vi "Q14070-Z040轴向间隙测试台1.vi"() -> ()   [LabVIEW 2013]
uses:
  <vilib>/printing/EasyPrintingControls.llb/report_type.ctl
  <vilib>/printing/EasyPrintingControls.llb/contents.ctl
  <vilib>/Utility/NIReport.llb/NI_report.lvclass
  <vilib>/Utility/file.llb/Write To Spreadsheet File (DBL).vi
  <vilib>/printing/EasyPrinting.llb/Easy Print VI Panel or Documentation (path).vi
  PCI8622_32.dll
  <vilib>/Utility/NIReport.llb/NI_ReportGenerationCore.lvlib
panel:
  in  "循环次数":u16
  out "左最大间隙值(mm)":dbl format="%#.6f"
  out "右最大间隙值(mm)":dbl format="%#.6f"
  out "旋转左极限位(mm)":dbl=-40.0
  out "旋转右极限位(mm)":dbl=60.0
  out "输入轴快进位置(mm)":dbl=-40.0
  out "输入轴初始位置(mm)":dbl=60.0
  out "输入轴最终位置（mm)":dbl format="%#.3f"
  out "左右基准":dbl=-40.0
  in  "进给速度":dbl=10.0
  in  "旋转速度":dbl=10.0
  out "DeviceHandle":u32
  out "输入轴电机慢进位置3":dbl format="%#.3f"
  out "输入轴电机慢进位置2":dbl format="%#.3f"
  out "旋转轴伺服位置":dbl=10000.0 format="%#.2f"
  out "复位按钮":bool=TRUE
  out "报警工步号":dbl
  out "报警信息":string
  out "输入轴伺服位置":dbl=10000.0 format="%#.1f"
  out "力矩（nm)":dbl format="%#.2f"
  out "位移(mm)":dbl format="%#.3f"
  in  "员工权限":bool
  out "测试操作状态":string
  out "测试 工步号":dbl
  out "通讯状态":bool
  in  "停止":bool
  out "流水线操作状态":string
  in  "流水线工步号":dbl
  in  "联线按钮":bool
  in  "选项卡控件 2":enum32{"间隙曲线", "手动", "传感器校验", "参数查询"}(tab)
  out "检测扭矩(NM)":dbl format="%#.1f"
  out "轴向间隙值(mm)":dbl format="%#.3f"
  out "本序完成":bool
  out "上序合格":bool
  out "上序完成":bool
  out "本序合格":bool
  out "间隙合格标准值(mm)":dbl=0.2
  out "换向扭矩(NM)":dbl format="%#.1f"
  out "XY图":cluster{dbl[], dbl[]}[](graph)
  in  "扳手无效":bool
  out "流水线气缸下限":bool
  out "流水线气缸上限":bool
  out "下工位检测":bool
  out "本工位检测":bool
  out "上工位检测":bool
  in  "M顶升气缸上升":bool
  in  "M顶升气缸下降":bool
  in  "M本阻挡器":bool
  in  "M上阻挡器":bool
  in  "电机回零":bool
  in  "电机下降":bool
  in  "电机上升":bool
  in  "左旋":bool
  in  "右旋":bool
  in  "扭矩传感器零点偏移":dbl format="%#.2f"
  in  "扭矩传感器比例偏移":dbl=1.0 format="%#.2f"
  in  "位移传感器零点偏移":dbl format="%#.2f"
  in  "位移传感器比例偏移":dbl=1.0 format="%#.2f"
  in  "传感器参数保存":bool
  in  "参数查询":bool
  in  "参数列表":string[][](table)
  in  "员工ID":string
  out "员工姓名":string
  in  "型号选择":u16(ring) items=["J706", "J709"]
  in  "参数加载":bool
  out "产品ID":string
  out "轴向间隙比例系数":dbl=1.0 format="%#_2f"
  out "error out 2":errorcluster
  out "输入轴电机快进速度":dbl format="%#.1f"
  out "输入轴电机慢进速度":dbl format="%#.3f"
  out "旋转电机速度":dbl=5.0 format="%#.3f"
  out "ADODB._Connection Out":refnum<k7>
  out "error out 3":errorcluster
  out "error out":errorcluster
  out "急停按钮":bool=TRUE
  out "芯片ID":string
  out "旋转轴AxisHandle OUT":u32
  out "FGCS":string
  out "RFID读取完成":bool
  out "RFID读取触发":bool
  out "Z040 RFID":string="A001"
  out "KSJJ":string
  out "ReturnValue 3":u32
  out "ReturnValue":u32
  out "输入轴AxisHandle OUT":u32
  out "产品选型":dbl
  # "Q14070-Z040  齿轮轴轴向间隙测试台"
  # "Q14070机械转向器装配线"
  # "Copying (C) 2015 湖北唯思凌科装备制造有限公司 版权所有"
  # "≤"
  # "传感器校验区"
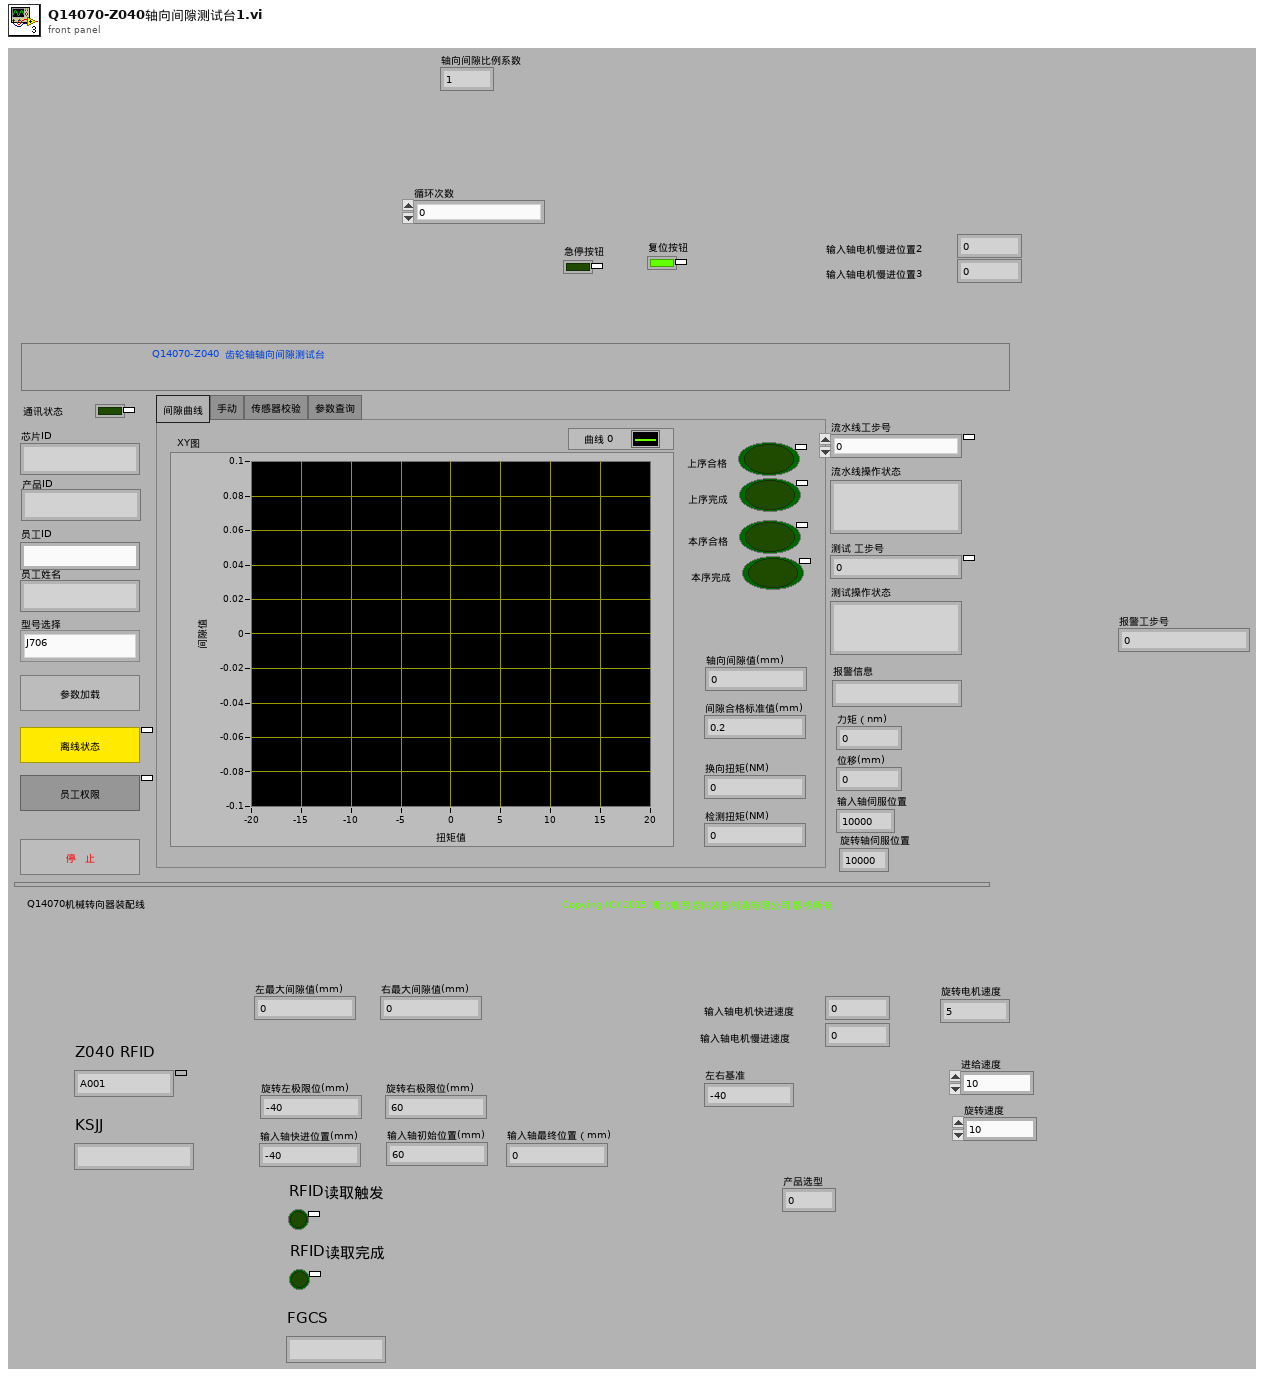
[diagram p1: front panel]
types:
  T1 = typedef "NI_ReportGenerationCore.lvlib/contents.ctl" = u16
  T2 = typedef "NI_ReportGenerationCore.lvlib/report_type.ctl" = u16
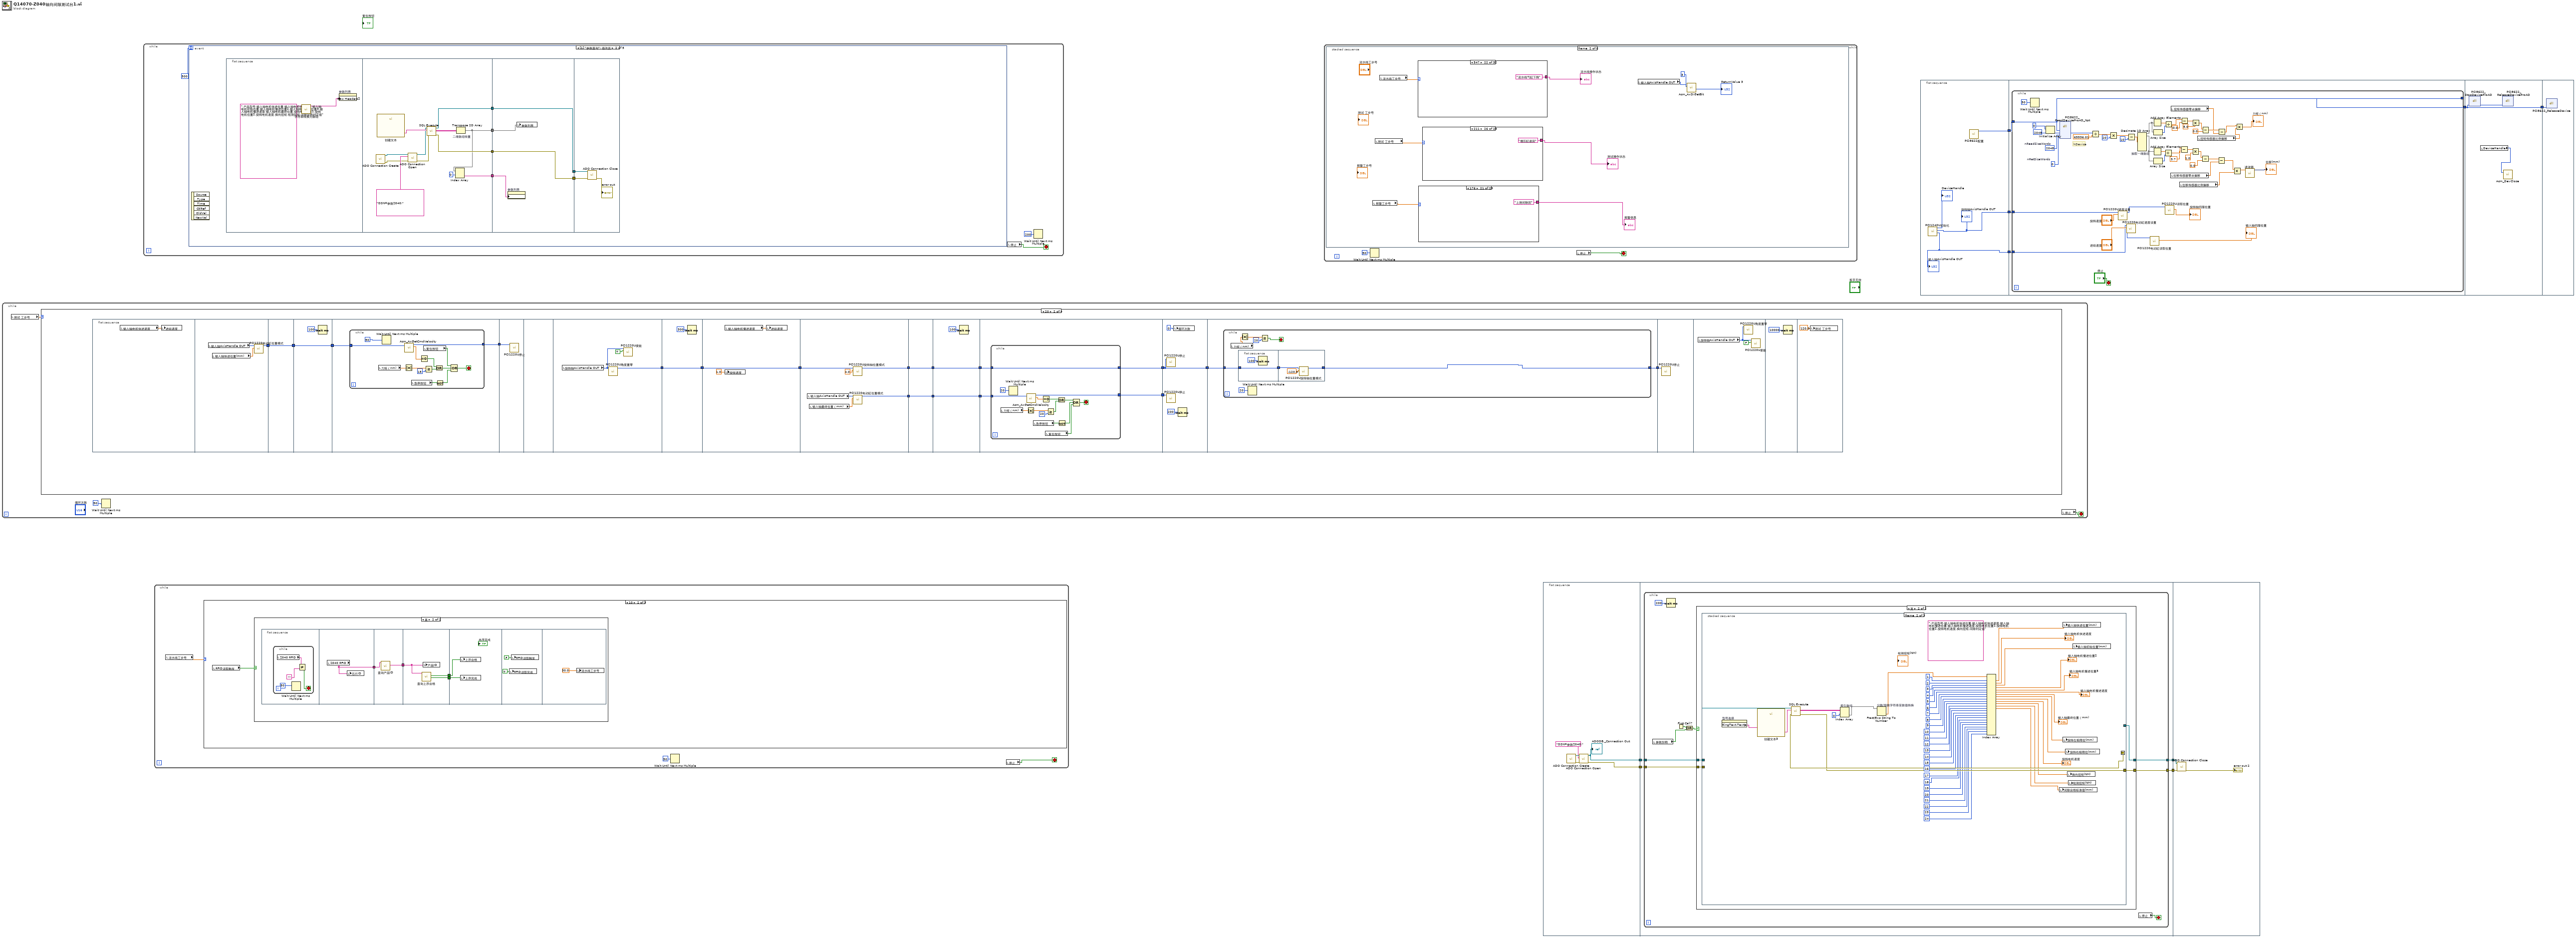
[diagram p0: block diagram]
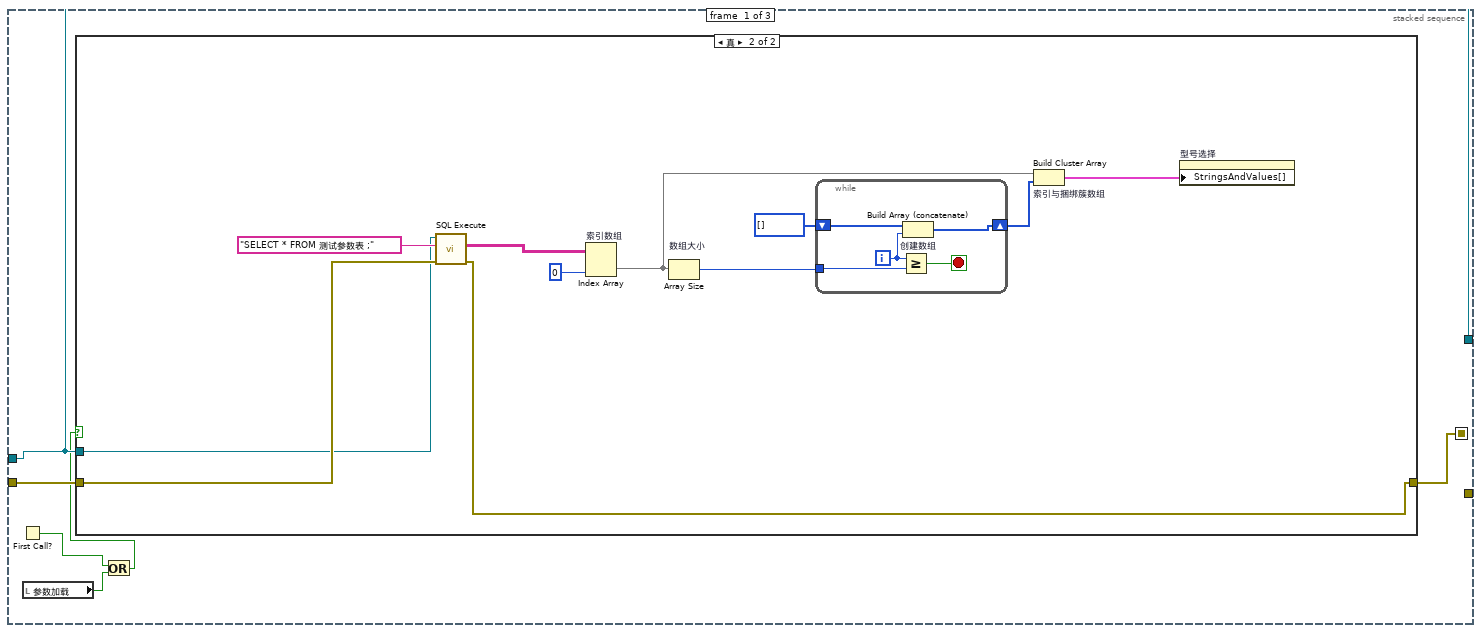
[diagram p3: hidden frame]
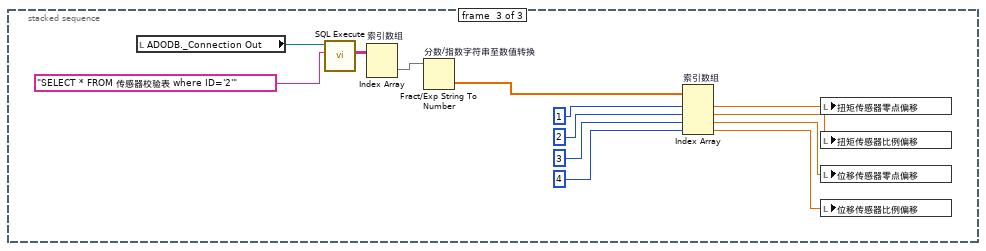
[diagram p5: hidden frame]
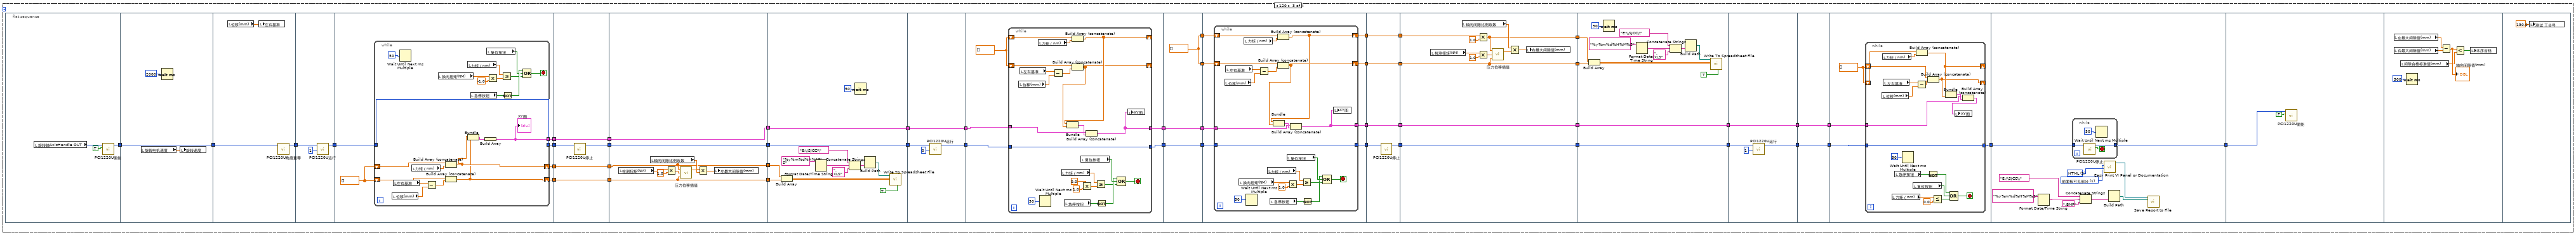
[diagram p7: hidden frame]
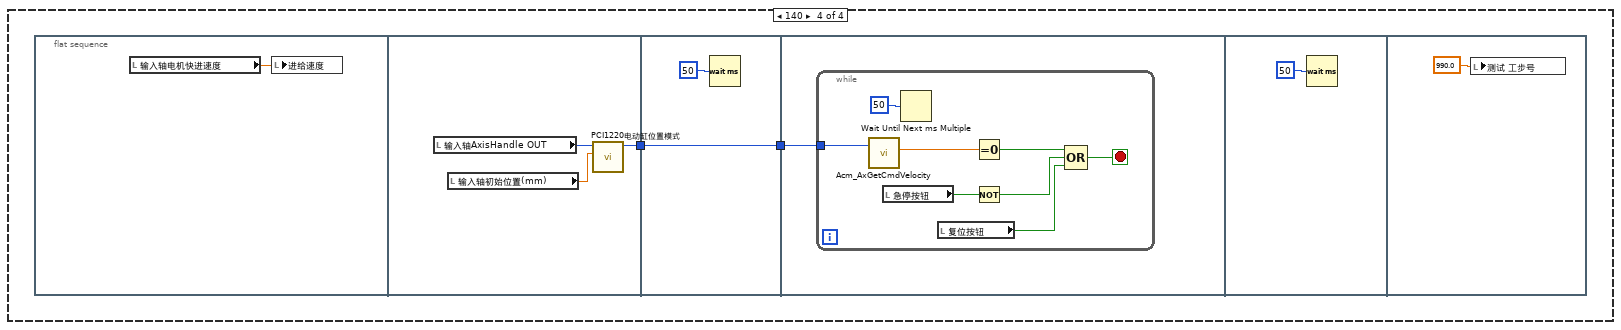
[diagram p8: hidden frame]
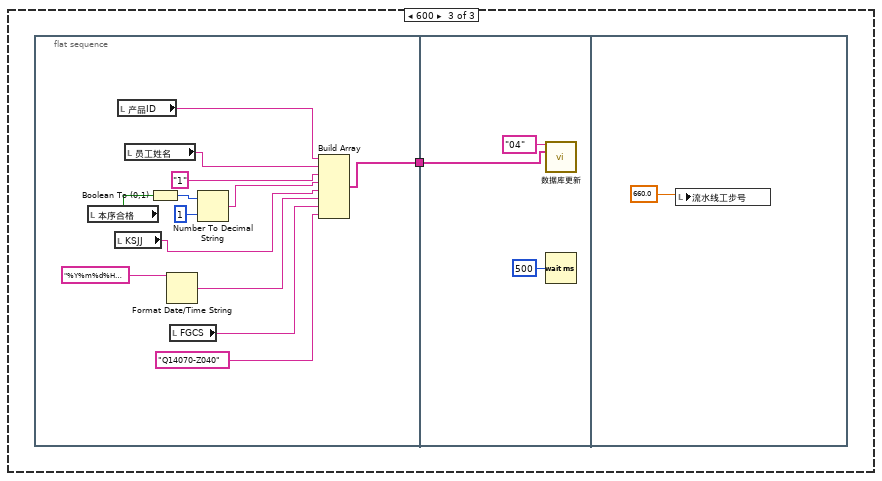
[diagram p11: hidden frame]
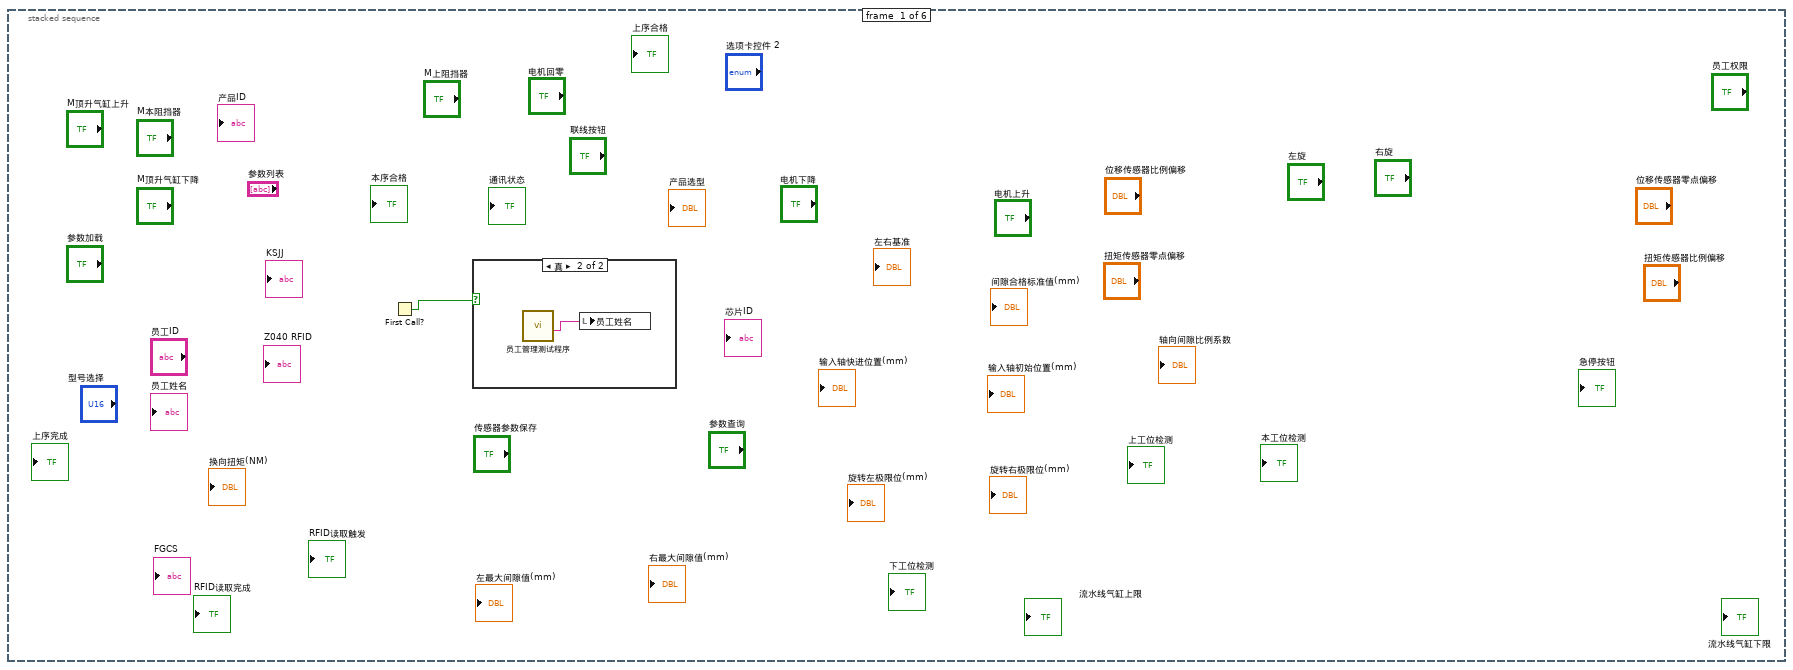
[diagram p12: hidden frame]
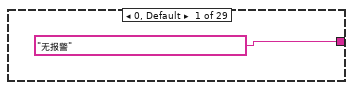
[diagram p14: hidden frame]
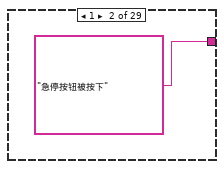
[diagram p15: hidden frame]
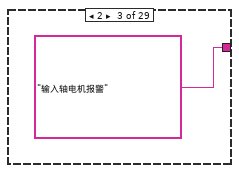
[diagram p16: hidden frame]
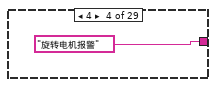
[diagram p17: hidden frame]
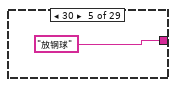
[diagram p18: hidden frame]
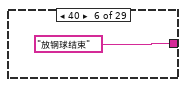
[diagram p19: hidden frame]
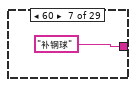
[diagram p20: hidden frame]
diagram:
  n1 = while {
    stop <- w10 stop-if-true
    n2 = local read "测试 工步号"() -> (w12:dbl)
    n3 = case shown="20" w12 {
      frame 0, Default {
      }
      frame 20 {
        n4 = flat-sequence {
          tunnel: [w33] -> w23
          tunnel: [w34] -> w27
          tunnel: w23 -> [w34]
          tunnel: w27 -> [w36]
          tunnel: [w36] -> w26
          tunnel: w26 -> [w38]
          tunnel: [w37] -> w29
          tunnel: w29 -> [w53]
          tunnel: [w55] -> w17
          tunnel: w17 -> [w58]
          tunnel: [w58] -> w16
          tunnel: w16 -> [w61]
          tunnel: [w61] -> w15
          tunnel: [w65] -> w22
          tunnel: w15 -> [w64]
          tunnel: [w62] -> w19
          tunnel: [w68] -> w25
          tunnel: w22 -> [w68]
          tunnel: [w69] -> w21
          tunnel: w19 -> [w69]
          tunnel: w25 -> [w72]
          tunnel: [w72] -> w24
          tunnel: w21 -> [w70]
          tunnel: [w70] -> w20
          tunnel: w24 -> [w76]
          tunnel: [w75] -> w28
          tunnel: w20 -> [w74]
          tunnel: [w73] -> w18
          tunnel: w28 -> [w95]
          tunnel: w18 -> [w93]
          tunnel: [w93] -> w14
          tunnel: w14 -> [w97]
          tunnel: [w96] -> w13
          tunnel: w13 -> [w111]
          frame #0 {
            n5 = local read "输入轴电机快进速度"() -> (w30:dbl)
            n6 = local write "进给速度"(w30) -> ()
          }
          frame #1 {
            n7 = local read "输入轴AxisHandle OUT"() -> (w31:u32)
            n8 = local read "输入轴快进位置(mm)"() -> (w32:dbl)
            n9 = call "PCI1220电动缸位置模式 .vi"("Distance"=w32, "AxisHandle IN"=w31) -> ("AxisHandle OUT"=w33:u32)  [unwired: 8 in, 1 out]
          }
          frame #2 {
          }
          frame #3 {
            n10 = Wait (ms)(milliseconds to wait=u32 100 ("等待时间（毫秒）")) -> ()  [unwired: 1 out]
          }
          frame #4 {
            n11 = while {
              tunnel: w38 -> [w49]
              tunnel: [w50] -> w37
              stop <- w40 stop-if-true
              n12 = local read "力矩（nm)"() -> (w47:dbl)
              n13 = Wait Until Next ms Multiple(millisecond multiple=u32 50 ("毫秒倍数")) -> ()  [unwired: 1 out]
              n14 = Absolute Value(x=w47) -> (abs(x)=w46:dbl)
              n15 = call <userlib>:"Acm_AxGetCmdVelocity.vi"("AxisHandle"=w49) -> ("Velocity"=w51:dbl, "AxisHandle"=w50:u32)  [unwired: 1 in, 2 out]
              n16 = local read "急停按钮"() -> (w43:bool)
              n17 = Equal To 0?(x=w51) -> (x = 0?=w48:bool)
              n18 = local read "复位按钮"() -> (w39:bool)
              n19 = Greater Or Equal?(x=w46, y=15) -> (x >= y?=w44:bool)
              n20 = Or(x=w48, y=w44) -> (x .or. y?=w42:bool)
              n21 = Not(x=w43) -> (.not. x?=w41:bool)
              n22 = Compound Arithmetic op=OR(w39, w42, w41) -> (w40:bool)
            }
          }
          frame #5 {
            n23 = call "PCI1220U停止.vi"("AxisHandle IN"=w53) -> ()  [unwired: 9 in, 2 out]
          }
          frame #6 {
          }
          frame #7 {
            n24 = local read "旋转轴AxisHandle OUT"() -> (w56:u32)
            n25 = call "PCI1220U角度置零.vi"("AxisHandle IN"=w56) -> ("AxisHandle OUT"=w55:u32)  [unwired: 10 in]
            n26 = call "PCI1220U使能.vi"("使能"=TRUE, "AxisHandle IN"=w56) -> ()  [unwired: 9 in, 1 out]
          }
          frame #8 {
            n27 = Wait (ms)(milliseconds to wait=u32 300 ("毫秒倍数")) -> ()  [unwired: 1 out]
          }
          frame #9 {
            n28 = local write "旋转速度"(1.0 ("旋转速度")) -> ()
            n29 = local read "输入轴电机慢进速度"() -> (w59:dbl)
            n30 = local write "进给速度"(w59) -> ()
          }
          frame #10 {
            n31 = local read "输入轴AxisHandle OUT"() -> (w67:u32)
            n32 = local read "输入轴最终位置（mm)"() -> (w66:dbl)
            n33 = call "PCI1220U旋转轴位置模式.vi"("Distance"=4.0, "AxisHandle IN"=w64) -> ("AxisHandle OUT"=w62:u32)  [unwired: 8 in, 1 out]
            n34 = call "PCI1220电动缸位置模式 .vi"("Distance"=w66, "AxisHandle IN"=w67) -> ("AxisHandle OUT"=w65:u32)  [unwired: 8 in, 1 out]
          }
          frame #11 {
          }
          frame #12 {
            n35 = Wait (ms)(milliseconds to wait=u32 100 ("等待时间（毫秒）")) -> ()  [unwired: 1 out]
          }
          frame #13 {
            n36 = while {
              tunnel: w76 -> [w90]
              tunnel: [w88] -> w75
              tunnel: w74 -> [w77]
              tunnel: [w77] -> w73
              stop <- w79 stop-if-true
              n37 = local read "力矩（nm)"() -> (w85:dbl)
              n38 = Wait Until Next ms Multiple(millisecond multiple=u32 20 ("毫秒倍数")) -> ()  [unwired: 1 out]
              n39 = Absolute Value(x=w85) -> (abs(x)=w86:dbl)
              n40 = call <userlib>:"Acm_AxGetCmdVelocity.vi"("AxisHandle"=w90) -> ("Velocity"=w89:dbl, "AxisHandle"=w88:u32)  [unwired: 1 in, 2 out]
              n41 = local read "急停按钮"() -> (w83:bool)
              n42 = Equal To 0?(x=w89) -> (x = 0?=w78:bool)
              n43 = local read "复位按钮"() -> (w80:bool)
              n44 = Greater Or Equal?(x=w86, y=20) -> (x >= y?=w84:bool)
              n45 = Or(x=w78, y=w84) -> (x .or. y?=w82:bool)
              n46 = Not(x=w83) -> (.not. x?=w81:bool)
              n47 = Compound Arithmetic op=OR(w82, w81, w80) -> (w79:bool)
            }
          }
          frame #14 {
            n48 = call "PCI1220U停止.vi"("AxisHandle IN"=w93) -> ()  [unwired: 9 in, 2 out]
            n49 = call "PCI1220U停止.vi"("AxisHandle IN"=w95) -> ()  [unwired: 9 in, 2 out]
            n50 = local write "循环次数"(u16 0 ("循环次数")) -> ()
            n51 = Wait (ms)(milliseconds to wait=u32 200 ("毫秒计时值")) -> ()  [unwired: 1 out]
          }
          frame #15 {
            n52 = while {
              tunnel: w97 -> [w99]
              tunnel: [w100] -> w96
              stop <- w102 stop-if-true
              n53 = local read "力矩（nm)"() -> (w101:dbl)
              n54 = flat-sequence {
                tunnel: w99 -> [w106]
                tunnel: [w106] -> w98
                tunnel: [w109] -> w100
                tunnel: w98 -> [w108]
                frame #0 {
                  n55 = Wait (ms)(milliseconds to wait=u32 100 ("等待时间（毫秒）")) -> ()  [unwired: 1 out]
                }
                frame #1 {
                  n56 = call "PCI1220U旋转轴位置模式.vi"("Distance"=-120.0, "AxisHandle IN"=w108) -> ("AxisHandle OUT"=w109:u32)  [unwired: 8 in, 1 out]
                }
              }
              n57 = Absolute Value(x=w101) -> (abs(x)=w103:dbl)
              n58 = Wait Until Next ms Multiple(millisecond multiple=u32 20 ("毫秒倍数")) -> ()  [unwired: 1 out]
              n59 = Greater Or Equal?(x=w103, y=20) -> (x >= y?=w102:bool)
            }
          }
          frame #16 {
            n60 = call "PCI1220U停止.vi"("AxisHandle IN"=w111) -> ()  [unwired: 9 in, 2 out]
          }
          frame #17 {
            n61 = local read "旋转轴AxisHandle OUT"() -> (w113:u32)
            n62 = call "PCI1220U角度置零.vi"("AxisHandle IN"=w113) -> ()  [unwired: 10 in, 1 out]
            n63 = call "PCI1220U使能.vi"("使能"=FALSE, "AxisHandle IN"=w113) -> ()  [unwired: 9 in, 1 out]
          }
          frame #18 {
            n64 = Wait (ms)(milliseconds to wait=u32 10000 ("等待时间（毫秒）")) -> ()  [unwired: 1 out]
          }
          frame #19 {
            n65 = local write "测试 工步号"(120.0 ("流水线工步号")) -> ()
          }
        }
      }
      frame 120 {
        n66 = flat-sequence {
          tunnel: [w162] -> w150
          tunnel: [w167] -> w151
          tunnel: w150 -> [w167]
          tunnel: w151 -> [w170]
          tunnel: [w169] -> w131
          tunnel: w131 -> [w172]
          tunnel: [w171] -> w139
          tunnel: w139 -> [w179]
          tunnel: [w178] -> w161
          tunnel: [w177] -> w160
          tunnel: [w176] -> w149
          tunnel: [w175] -> w128
          tunnel: w161 -> [w205]
          tunnel: w160 -> [w204]
          tunnel: [w204] -> w159
          tunnel: [w203] -> w158
          tunnel: [w202] -> w157
          tunnel: w149 -> [w203]
          tunnel: w128 -> [w201]
          tunnel: [w201] -> w127
          tunnel: w159 -> [w207]
          tunnel: w158 -> [w208]
          tunnel: w157 -> [w215]
          tunnel: [w215] -> w135
          tunnel: [w208] -> w133
          tunnel: [w207] -> w132
          tunnel: w127 -> [w206]
          tunnel: [w206] -> w126
          tunnel: w135 -> [w228]
          tunnel: [w228] -> w134
          tunnel: w133 -> [w220]
          tunnel: w132 -> [w219]
          tunnel: [w217] -> w130
          tunnel: w126 -> [w217]
          tunnel: w134 -> [w231]
          tunnel: [w230] -> w125
          tunnel: w130 -> [w229]
          tunnel: [w229] -> w123
          tunnel: w125 -> [w237]
          tunnel: [w234] -> w124
          tunnel: w123 -> [w236]
          tunnel: [w235] -> w122
          tunnel: [w262] -> w153
          tunnel: [w260] -> w152
          tunnel: [w260] -> w142
          tunnel: w124 -> [w262]
          tunnel: [w261] -> w129
          tunnel: w122 -> [w261]
          tunnel: w153 -> [w270]
          tunnel: w152 -> [w268]
          tunnel: [w269] -> w156
          tunnel: [w266] -> w155
          tunnel: [w265] -> w154
          tunnel: w142 -> [w267]
          tunnel: w129 -> [w264]
          tunnel: [w263] -> w121
          tunnel: w156 -> [w297]
          tunnel: w155 -> [w296]
          tunnel: [w296] -> w138
          tunnel: w154 -> [w295]
          tunnel: [w295] -> w137
          tunnel: [w294] -> w136
          tunnel: w121 -> [w293]
          tunnel: [w293] -> w120
          tunnel: w138 -> [w302]
          tunnel: w137 -> [w304]
          tunnel: [w307] -> w147
          tunnel: w136 -> [w307]
          tunnel: [w303] -> w141
          tunnel: [w302] -> w140
          tunnel: w120 -> [w298]
          tunnel: [w298] -> w119
          tunnel: [w322] -> w148
          tunnel: w147 -> [w322]
          tunnel: w141 -> [w315]
          tunnel: w140 -> [w314]
          tunnel: w119 -> [w310]
          tunnel: [w310] -> w118
          tunnel: w148 -> [w325]
          tunnel: [w324] -> w145
          tunnel: w118 -> [w323]
          tunnel: [w323] -> w117
          tunnel: [w328] -> w146
          tunnel: w145 -> [w328]
          tunnel: w117 -> [w327]
          tunnel: [w327] -> w116
          tunnel: w146 -> [w332]
          tunnel: [w331] -> w144
          tunnel: w116 -> [w329]
          tunnel: w144 -> [w363]
          tunnel: [w362] -> w143
          tunnel: w143 -> [w368]
          frame #0 {
            n67 = local read "旋转轴AxisHandle OUT"() -> (w164:u32)
            n68 = call "PCI1220U使能.vi"("使能"=TRUE, "AxisHandle IN"=w164) -> ("AxisHandle OUT"=w162:u32)  [unwired: 9 in]
          }
          frame #1 {
            n69 = local read "旋转电机速度"() -> (w166:dbl)
            n70 = Wait (ms)(milliseconds to wait=u32 2000 ("毫秒倍数")) -> ()  [unwired: 1 out]
            n71 = local write "旋转速度"(w166) -> ()
          }
          frame #2 {
            n72 = local read "位移(mm)"() -> (w168:dbl)
            n73 = local write "左右基准"(w168) -> ()
            n74 = call "PCI1220U角度置零.vi"("AxisHandle IN"=w170) -> ("AxisHandle OUT"=w169:u32)  [unwired: 10 in]
          }
          frame #3 {
            n75 = call "PCI1220U运行.vi"("方向"=u16 1, "AxisHandle IN"=w172) -> ("AxisHandle OUT"=w171:u32)  [unwired: 9 in]
          }
          frame #4 {
            w174 = dbl[] [] ("添加的数组")
            n76 = while {
              tunnel: w179 -> [w193]
              tunnel: [w193] -> w178
              shift-right: [w182] -> w176
              shift-left: w174 -> [w183]
              shift-right: [w181] -> w177
              shift-left: w174 -> [w187]
              tunnel: [w180] -> w175
              stop <- w188 stop-if-true
              n77 = local read "位移(mm)"() -> (w186:dbl)
              n78 = local read "左右基准"() -> (w185:dbl)
              n79 = Wait Until Next ms Multiple(millisecond multiple=u32 50 ("毫秒倍数")) -> ()  [unwired: 1 out]
              n80 = local read "力矩（nm)"() -> (w200:dbl)
              n81 = Subtract(x=w185, y=w186) -> (x-y=w198:dbl)
              n82 = local read "换向扭矩(NM)"() -> (w197:dbl)
              n83 = Build Array (concatenate)(w183, w200) -> (w182:dbl[])
              n84 = Build Array (concatenate)(w187, w198) -> (w181:dbl[])
              n85 = Bundle(w182, w181) -> (w184:cluster{dbl[], dbl[]})  [unwired: 1 in]
              n86 = local read "力矩（nm)"() -> (w195:dbl)
              n87 = local read "急停按钮"() -> (w192:bool)
              n88 = Build Array(w184) -> (w180:cluster{dbl[], dbl[]}[])
              "XY图" <- w180
              n89 = local read "复位按钮"() -> (w190:bool)
              n90 = Multiply(x=w197, y=-1.0) -> (x*y=w194:dbl)
              n91 = Less Or Equal?(x=w195, y=w194) -> (x <= y?=w189:bool)
              n92 = Not(x=w192) -> (.not. x?=w191:bool)
              n93 = Compound Arithmetic op=OR(w191, w190, w189) -> (w188:bool)
            }
          }
          frame #5 {
            n94 = call "PCI1220U停止.vi"("AxisHandle IN"=w205) -> ("AxisHandle OUT"=w202:u32)  [unwired: 9 in, 1 out]
          }
          frame #6 {
            n95 = local read "检测扭矩(NM)"() -> (w209:dbl)
            n96 = local read "轴向间隙比例系数"() -> (w212:dbl)
            n97 = Multiply(x=w209, y=1.0) -> (x*y=w211:dbl)
            n98 = call "压力位移插值.vi"("压力数组"=w207, "监控点位移"=w211, "位移数组"=w208) -> ("监控点压力"=w213:dbl)  [unwired: 2 in]
            n99 = Multiply(x=w212, y=w213) -> (x*y=w214:dbl)
            n100 = local write "左最大间隙值(mm)"(w214) -> ()
          }
          frame #7 {
            n101 = Build Array(w220, w219) -> (w218:dbl[][])
            n102 = Format Date/Time String(time format string (%c)="%y%m%d%H%M%S" ("时间格式字符串(%c)")) -> (date/time string=w227:string)  [unwired: 2 in]
            n103 = Concatenate Strings("E:\\SJCC\\" ("时间格式字符串(%c)"), w227, ".XLS") -> (w222:string)
            n104 = Wait (ms)(milliseconds to wait=u32 50 ("等待时间（毫秒）")) -> ()  [unwired: 1 out]
            n105 = Build Path(name or relative path=w222) -> (appended path=w223:path)  [unwired: 1 in]
            n106 = call-poly <vilib>:"Write To Spreadsheet File.vi"("transpose? (no:F)"=TRUE, "2D data"=w218, "file path (dialog if empty)"=w223) -> ()  [unwired: 5 in, 1 out]
          }
          frame #8 {
            n107 = call "PCI1220U运行.vi"("方向"=u16 0, "AxisHandle IN"=w231) -> ("AxisHandle OUT"=w230:u32)  [unwired: 9 in]
          }
          frame #9 {
            w233 = dbl[] [] ("添加的数组")
            n108 = while {
              tunnel: w237 -> [w254]
              tunnel: [w254] -> w234
              shift-right: [w243] -> _
              shift-left: w233 -> [w248]
              shift-right: [w242] -> _
              shift-left: w233 -> [w247]
              tunnel: w236 -> [w239]
              tunnel: [w241] -> w235
              stop <- w249 stop-if-true
              n109 = local read "位移(mm)"() -> (w245:dbl)
              n110 = local read "左右基准"() -> (w244:dbl)
              n111 = local read "力矩（nm)"() -> (w259:dbl)
              n112 = Wait Until Next ms Multiple(millisecond multiple=u32 50 ("毫秒倍数")) -> ()  [unwired: 1 out]
              n113 = Subtract(x=w244, y=w245) -> (x-y=w246:dbl)
              n114 = local read "力矩（nm)"() -> (w257:dbl)
              n115 = local read "急停按钮"() -> (w251:bool)
              n116 = Build Array (concatenate)(w248, w259) -> (w243:dbl[])
              n117 = Build Array (concatenate)(w247, w246) -> (w242:dbl[])
              n118 = Bundle(w243, w242) -> (w238:cluster{dbl[], dbl[]})  [unwired: 1 in]
              n119 = local read "复位按钮"() -> (w253:bool)
              n120 = Multiply(x=0.0, y=1.0) -> (x*y=w255:dbl)
              n121 = Build Array (concatenate)(w239, w238) -> (w241:cluster{dbl[], dbl[]}[])
              n122 = Greater Or Equal?(x=w257, y=w255) -> (x >= y?=w250:bool)
              n123 = Not(x=w251) -> (.not. x?=w252:bool)
              n124 = Compound Arithmetic op=OR(w252, w253, w250) -> (w249:bool)
              n125 = local write "XY图"(w241) -> ()
            }
          }
          frame #10 {
            w260 = dbl[] [] ("添加的数组")
          }
          frame #11 {
            n126 = while {
              tunnel: w270 -> [w286]
              tunnel: [w286] -> w269
              shift-right: [w275] -> w265
              shift-left: w268 -> [w280]
              shift-right: [w274] -> w266
              shift-left: w267 -> [w279]
              tunnel: w264 -> [w271]
              tunnel: [w273] -> w263
              stop <- w281 stop-if-true
              n127 = local read "位移(mm)"() -> (w277:dbl)
              n128 = local read "左右基准"() -> (w276:dbl)
              n129 = local read "换向扭矩(NM)"() -> (w289:dbl)
              n130 = local read "力矩（nm)"() -> (w292:dbl)
              n131 = Wait Until Next ms Multiple(millisecond multiple=u32 50 ("毫秒倍数")) -> ()  [unwired: 1 out]
              n132 = Subtract(x=w276, y=w277) -> (x-y=w278:dbl)
              n133 = local read "力矩（nm)"() -> (w290:dbl)
              n134 = local read "急停按钮"() -> (w283:bool)
              n135 = Build Array (concatenate)(w280, w292) -> (w275:dbl[])
              n136 = Build Array (concatenate)(w279, w278) -> (w274:dbl[])
              n137 = Bundle(w275, w274) -> (w272:cluster{dbl[], dbl[]})  [unwired: 1 in]
              n138 = local read "复位按钮"() -> (w285:bool)
              n139 = Multiply(x=w289, y=1.0) -> (x*y=w287:dbl)
              n140 = Build Array (concatenate)(w271, w272) -> (w273:cluster{dbl[], dbl[]}[])
              n141 = Greater Or Equal?(x=w290, y=w287) -> (x >= y?=w282:bool)
              n142 = Not(x=w283) -> (.not. x?=w284:bool)
              n143 = Compound Arithmetic op=OR(w284, w285, w282) -> (w281:bool)
              n144 = local write "XY图"(w273) -> ()
            }
          }
          frame #12 {
            n145 = call "PCI1220U停止.vi"("AxisHandle IN"=w297) -> ("AxisHandle OUT"=w294:u32)  [unwired: 9 in, 1 out]
          }
          frame #13 {
            n146 = local read "检测扭矩(NM)"() -> (w301:dbl)
            n147 = local read "轴向间隙比例系数"() -> (w309:dbl)
            n148 = Multiply(x=w304, y=1.0) -> (x*y=w303:dbl[])
            n149 = Multiply(x=w301, y=1.0) -> (x*y=w300:dbl)
            n150 = call "压力位移插值.vi"("压力数组"=w302, "监控点位移"=w300, "位移数组"=w303) -> ("监控点压力"=w306:dbl)  [unwired: 2 in]
            n151 = Multiply(x=w309, y=w306) -> (x*y=w308:dbl)
            n152 = local write "右最大间隙值(mm)"(w308) -> ()
          }
          frame #14 {
            n153 = Build Array(w315, w314) -> (w316:dbl[][])
            n154 = Wait (ms)(milliseconds to wait=u32 50 ("等待时间（毫秒）")) -> ()  [unwired: 1 out]
            n155 = Format Date/Time String(time format string (%c)="%y%m%d%H%M%S" ("时间格式字符串(%c)")) -> (date/time string=w312:string)  [unwired: 2 in]
            n156 = Concatenate Strings("E:\\SJCC\\" ("时间格式字符串(%c)"), w312, ".XLS") -> (w320:string)
            n157 = Build Path(name or relative path=w320) -> (appended path=w319:path)  [unwired: 1 in]
            n158 = call-poly <vilib>:"Write To Spreadsheet File.vi"("transpose? (no:F)"=TRUE, "2D data"=w316, "file path (dialog if empty)"=w319) -> ()  [unwired: 5 in, 1 out]
          }
          frame #15 {
            n159 = call "PCI1220U运行.vi"("方向"=u16 1, "AxisHandle IN"=w325) -> ("AxisHandle OUT"=w324:u32)  [unwired: 9 in]
          }
          frame #16 {
          }
          frame #17 {
            w330 = dbl[] [] ("添加的数组")
            n160 = while {
              tunnel: w332 -> [w350]
              tunnel: [w350] -> w331
              shift-right: [w334] -> _
              shift-left: w330 -> [w339]
              shift-right: [w333] -> _
              shift-left: w330 -> [w338]
              tunnel: w329 -> [w335]
              stop <- w345 stop-if-true
              n161 = local read "位移(mm)"() -> (w342:dbl)
              n162 = local read "力矩（nm)"() -> (w340:dbl)
              n163 = local read "左右基准"() -> (w343:dbl)
              n164 = local read "力矩（nm)"() -> (w351:dbl)
              n165 = local read "急停按钮"() -> (w347:bool)
              n166 = Wait Until Next ms Multiple(millisecond multiple=u32 50 ("毫秒倍数")) -> ()  [unwired: 1 out]
              n167 = local read "复位按钮"() -> (w349:bool)
              n168 = Build Array (concatenate)(w339, w340) -> (w334:dbl[])
              n169 = Subtract(x=w343, y=w342) -> (x-y=w341:dbl)
              n170 = Not(x=w347) -> (.not. x?=w348:bool)
              n171 = Build Array (concatenate)(w338, w341) -> (w333:dbl[])
              n172 = Less Or Equal?(x=w351, y=0.0) -> (x <= y?=w346:bool)
              n173 = Bundle(w334, w333) -> (w336:cluster{dbl[], dbl[]})  [unwired: 1 in]
              n174 = Compound Arithmetic op=OR(w348, w349, w346) -> (w345:bool)
              n175 = Build Array (concatenate)(w335, w336) -> (w337:cluster{dbl[], dbl[]}[])
              n176 = local write "XY图"(w337) -> ()
            }
          }
          frame #18 {
            w359 = T1 1 items=["完整前面板", "前面板可见部分", "图标、说明、前面板和程序框图", "说明信息：使用前面板", "说明信息：作为子VI使用", "说明信息：完整", "说明信息：自定义"] ("contents (complete front panel)")
            w361 = T2 2 items=["快速打印", "标准报表", "HTML", "双字节", "Excel"] ("report type (Quick Print)")
            n177 = Format Date/Time String(time format string (%c)="%y%m%d%H%M%S" ("时间格式字符串(%c)")) -> (date/time string=w354:string)  [unwired: 2 in]
            n178 = while {
              tunnel: w363 -> [w367]
              tunnel: [w364] -> w362
              stop <- w366 stop-if-true
              n179 = call "PCI1220U停止.vi"("AxisHandle IN"=w367) -> ("完成"=w366:bool, "AxisHandle OUT"=w364:u32)  [unwired: 9 in]
              n180 = Wait Until Next ms Multiple(millisecond multiple=u32 50 ("毫秒倍数")) -> ()  [unwired: 1 out]
            }
            n181 = Concatenate Strings("E:\\SJCC\\" ("时间格式字符串(%c)"), w354, ".BMP" ("产品ID")) -> (w360:string)
            n182 = call-poly <vilib>:"Easy Print VI Panel or Documentation.vi"("report type (Quick Print)"=w361, "contents (complete front panel)"=w359) -> ("report out"=w353:refnum<class "NI_report.lvclass">)  [unwired: 8 in, 1 out]
            n183 = Build Path(name or relative path=w360) -> (appended path=w357:path)  [unwired: 1 in]
            n184 = call-dynamic "Save Report to File.vi"("report in"=w353, "report file path"=w357) -> ()  [unwired: 12 in, 2 out]
          }
          frame #19 {
            n185 = call "PCI1220U使能.vi"("使能"=FALSE, "AxisHandle IN"=w368) -> ()  [unwired: 9 in, 1 out]
          }
          frame #20 {
            n186 = local read "左最大间隙值(mm)"() -> (w371:dbl)
            n187 = local read "右最大间隙值(mm)"() -> (w370:dbl)
            n188 = local read "间隙合格标准值(mm)"() -> (w373:dbl)
            n189 = Wait (ms)(milliseconds to wait=u32 500 ("等待时间（毫秒）")) -> ()  [unwired: 1 out]
            n190 = Subtract(x=w371, y=w370) -> (x-y=w375:dbl)
            "轴向间隙值(mm)" <- w375
            n191 = Less?(x=w375, y=w373) -> (x < y?=w374:bool)
            n192 = local write "本序合格"(w374) -> ()
          }
          frame #21 {
            n193 = local write "测试 工步号"(130.0 ("测试 工步号")) -> ()
          }
        }
      }
      frame 140 {
        n194 = flat-sequence {
          tunnel: [w381] -> w377
          tunnel: [w383] -> w378
          tunnel: w377 -> [w383]
          tunnel: w378 -> [w385]
          frame #0 {
            n195 = local read "输入轴电机快进速度"() -> (w379:dbl)
            n196 = local write "进给速度"(w379) -> ()
          }
          frame #1 {
            n197 = local read "输入轴AxisHandle OUT"() -> (w382:u32)
            n198 = local read "输入轴初始位置(mm)"() -> (w380:dbl)
            n199 = call "PCI1220电动缸位置模式 .vi"("Distance"=w380, "AxisHandle IN"=w382) -> ("AxisHandle OUT"=w381:u32)  [unwired: 8 in, 1 out]
          }
          frame #2 {
            n200 = Wait (ms)(milliseconds to wait=u32 50 ("毫秒倍数")) -> ()  [unwired: 1 out]
          }
          frame #3 {
            n201 = while {
              tunnel: w385 -> [w392]
              stop <- w386 stop-if-true
              n202 = call <userlib>:"Acm_AxGetCmdVelocity.vi"("AxisHandle"=w392) -> ("Velocity"=w391:dbl)  [unwired: 1 in, 3 out]
              n203 = local read "急停按钮"() -> (w390:bool)
              n204 = Wait Until Next ms Multiple(millisecond multiple=u32 50 ("毫秒倍数")) -> ()  [unwired: 1 out]
              n205 = local read "复位按钮"() -> (w387:bool)
              n206 = Equal To 0?(x=w391) -> (x = 0?=w389:bool)
              n207 = Not(x=w390) -> (.not. x?=w388:bool)
              n208 = Compound Arithmetic op=OR(w389, w388, w387) -> (w386:bool)
            }
          }
          frame #4 {
            n209 = Wait (ms)(milliseconds to wait=u32 50 ("毫秒倍数")) -> ()  [unwired: 1 out]
          }
          frame #5 {
            n210 = local write "测试 工步号"(990.0 ("测试 工步号")) -> ()
          }
        }
      }
    }
    n211 = Wait Until Next ms Multiple(millisecond multiple=u32 50 ("毫秒倍数")) -> ()  [unwired: 1 out]
    n212 = local read "停止"() -> (w10:bool)
  }
  n213 = while {
    stop <- w396 stop-if-true
    n214 = event shown="[1] \"参数查询\": 值改变" {
      selector: _ -> [_ _ _ _ _]
      dyn-events: _ -> [_ _ _ _ _]
      timeout: 500 -> [_ _ _ _ _]
      event Timeout {
        n215 = event-data() -> ()  [unwired: 3 out]
      }
      event "参数查询": Value Change {
        n216 = event-data() -> ()  [unwired: 7 out]
        n217 = flat-sequence {
          tunnel: [w407] -> w404
          tunnel: [w417] -> w403
          tunnel: [w413] -> w402
          tunnel: [w410] -> w401
          tunnel: w404 -> [w422]
          tunnel: w403 -> [w420]
          tunnel: [w421] -> w400
          tunnel: w402 -> [w421]
          tunnel: [w420] -> w399
          tunnel: w401 -> [w419]
          tunnel: w400 -> [w425]
          tunnel: w399 -> [w424]
          frame #0 {
            n218 = call "字符串转换为数组.vi"("查询内容"=",产品型号,输入轴电机快进位置,输入轴电机快进速度,输入轴电机初始位置,输入轴电机慢进位置2,输入轴电机慢进位置3,输入轴电机慢进速度,输入轴电机最终位置,旋转电机位置1,旋转电机位置2,旋转电机速度,换向扭矩,检测扭矩,间隙合格判定值") -> ("列首"=w405:string[])  [unwired: 10 in]
            n219 = property on="参数列表" class="Tbl (严格)"("Row Headers[]"=w405) -> ()  [unwired: 2 in, 2 out]
          }
          frame #1 {
            n220 = call "ADO Connection Create.vi"() -> ("error out"=w412:errorcluster, "ADODB._Connection Out"=w416:refnum<k7>)  [unwired: 10 in]
            n221 = call "创建文本"() -> ("Result"=w418:string)  [unwired: 14 in, 1 out]
            n222 = call "ADO Connection Open.vi"("error in (no error)"=w412, "ConnectionString"="DSN=参数Z040;", "ADODB._Connection In"=w416) -> ("error out"=w411:errorcluster, "ADODB._Connection Out"=w414:refnum<k7>)  [unwired: 7 in]
            n223 = call "SQL Execute.vi"("error in (no error)"=w411, "Command Text"=w418, "ADODB._Connection In"=w414) -> ("error out"=w417:errorcluster, "Data"=w409:string[][], "ADODB._Connection Out"=w413:refnum<k7>)  [unwired: 5 in, 1 out]
            n224 = Transpose 2D Array "二维数组转置"(2D array=w409) -> (transposed array=w407:string[][])
            n225 = Index Array(array=w407, index (row)=0 ("索引 (行)")) -> (element=w410:string[])  [unwired: 1 in]
          }
          frame #2 {
            n226 = property on="参数列表" class="Tbl (严格)"("Column Headers[]"=w419) -> ()  [unwired: 2 in, 2 out]
            n227 = local write "参数列表"(w422) -> ()
          }
          frame #3 {
            n228 = call "ADO Connection Close.vi"("error in (no error)"=w424, "ADODB._Connection In"=w425) -> ("error out"=→"error out":errorcluster)  [unwired: 8 in, 1 out]
          }
        }
      }
      event "传感器参数保存": Value Change {
        n229 = event-data() -> ()  [unwired: 7 out]
        n230 = local read "位移传感器比例偏移"() -> (w426:dbl)
        n231 = local read "位移传感器零点偏移"() -> (w427:dbl)
        n232 = local read "扭矩传感器比例偏移"() -> (w428:dbl)
        n233 = local read "扭矩传感器零点偏移"() -> (w429:dbl)
        n234 = Number To Fractional String(number=w427, precision (6)=i16 1 ("精度(6)")) -> (F-format string=w433:string)  [unwired: 2 in]
        n235 = Number To Fractional String(number=w428, precision (6)=i16 2 ("精度(6)")) -> (F-format string=w434:string)  [unwired: 2 in]
        n236 = Number To Fractional String(number=w429, precision (6)=i16 3 ("精度(6)")) -> (F-format string=w435:string)  [unwired: 2 in]
        n237 = Number To Fractional String(number=w426, precision (6)=i16 2 ("精度(6)")) -> (F-format string=w432:string)  [unwired: 2 in]
        n238 = call "创建文本2"("位移1比例偏移值"=w432, "压力1零点偏移值"=w435, "压力1比例偏移值"=w434, "位移1零点偏移值"=w433) -> ("Result"=w431:string)  [unwired: 10 in, 1 out]
        n239 = call "ADO Connection Create.vi"() -> ("error out"=w442:errorcluster, "ADODB._Connection Out"=w444:refnum<k7>)  [unwired: 10 in]
        n240 = call "ADO Connection Open.vi"("error in (no error)"=w442, "ConnectionString"="DSN=参数Z040;", "ADODB._Connection In"=w444) -> ("error out"=w441:errorcluster, "ADODB._Connection Out"=w443:refnum<k7>)  [unwired: 7 in]
        n241 = call "SQL Execute.vi"("error in (no error)"=w441, "Command Text"=w431, "ADODB._Connection In"=w443) -> ("error out"=w445:errorcluster, "ADODB._Connection Out"=w446:refnum<k7>)  [unwired: 5 in, 2 out]
        n242 = call "ADO Connection Close.vi"("error in (no error)"=w445, "ADODB._Connection In"=w446) -> ("error out"=→"error out 3":errorcluster)  [unwired: 8 in, 1 out]
      }
      event "停止": Value Change {
        n243 = event-data() -> ()  [unwired: 7 out]
        n244 = flat-sequence {
          frame #0 {
            n245 = local write "流水线工步号"(0.0 ("工步号")) -> ()
          }
          frame #1 {
            n246 = Wait Until Next ms Multiple(millisecond multiple=u32 1000 ("毫秒倍数")) -> ()  [unwired: 1 out]
          }
          frame #2 {
            n247 = Quit LabVIEW(quit? (T)=TRUE ("停止？(T)")) -> ()
          }
        }
      }
      event "电机回零": Mouse Down {
        n248 = event-data() -> ()  [unwired: 9 out]
        n249 = flat-sequence {
          tunnel: [w458] -> w454
          tunnel: w454 -> [w461]
          tunnel: [w461] -> w453
          tunnel: w453 -> [w463]
          tunnel: [w463] -> w452
          tunnel: w452 -> [w464]
          tunnel: [w464] -> w451
          tunnel: [w465] -> w456
          tunnel: w451 -> [w466]
          tunnel: w456 -> [w471]
          tunnel: [w471] -> w455
          tunnel: w455 -> [w473]
          tunnel: [w473] -> w457
          tunnel: [w472] -> w450
          tunnel: w457 -> [w484]
          tunnel: w450 -> [w483]
          frame #0 {
            n250 = local read "输入轴AxisHandle OUT"() -> (w458:u32)
            n251 = call "PCI1220U使能.vi"("使能"=TRUE, "AxisHandle IN"=w458) -> ()  [unwired: 9 in, 1 out]
          }
          frame #1 {
            n252 = Wait Until Next ms Multiple(millisecond multiple=u32 50 ("毫秒倍数")) -> ()  [unwired: 1 out]
          }
          frame #2 {
            n253 = local write "进给速度"(10.0 ("进给速度")) -> ()
          }
          frame #3 {
          }
          frame #4 {
            n254 = call <userlib>:"Acm_AxHome.vi"("DirMode"=u32 1, "HomeMode"=u32 11, "AxisHandle"=w466) -> ("ReturnValue"=→"ReturnValue":u32, "AxisHandle"=w465:u32)  [unwired: 1 in, 1 out]
          }
          frame #5 {
            n255 = Wait (ms)(milliseconds to wait=u32 100 ("等待时间（毫秒）")) -> ()  [unwired: 1 out]
          }
          frame #6 {
            n256 = while {
              tunnel: w473 -> [w482]
              tunnel: [w474] -> w472
              stop <- w475 stop-if-true
              n257 = local read "急停按钮"() -> (w479:bool)
              n258 = local read "复位按钮"() -> (w476:bool)
              n259 = call <userlib>:"Acm_AxGetCmdVelocity.vi"("AxisHandle"=w482) -> ("Velocity"=w481:dbl, "AxisHandle"=w474:u32)  [unwired: 1 in, 2 out]
              n260 = Equal To 0?(x=w481) -> (x = 0?=w478:bool)
              n261 = Not(x=w479) -> (.not. x?=w477:bool)
              n262 = Wait Until Next ms Multiple(millisecond multiple=u32 50 ("毫秒倍数")) -> ()  [unwired: 1 out]
              n263 = Compound Arithmetic op=OR(w478, w477, w476) -> (w475:bool)
            }
          }
          frame #7 {
            n264 = call "PCI1220U角度置零.vi"("AxisHandle IN"=w484) -> ()  [unwired: 10 in, 1 out]
            n265 = call "PCI1220U停止.vi"("AxisHandle IN"=w483) -> ()  [unwired: 9 in, 2 out]
          }
          frame #8 {
            n266 = local write "电机回零"(FALSE ("回零")) -> ()
          }
        }
      }
    }
    n267 = local read "停止"() -> (w396:bool)
    n268 = Wait Until Next ms Multiple(millisecond multiple=u32 200 ("毫秒倍数")) -> ()  [unwired: 1 out]
  }
  n269 = while {
    stop <- w488 stop-if-true
    n270 = local read "流水线工步号"() -> (w486:dbl)
    n271 = case shown="10" w486 {
      frame 0, Default {
      }
      frame 10 {
        n272 = local read "RFID读取触发"() -> (w489:bool)
        n273 = case shown="真" w489 {
          frame False {
          }
          frame True {
            n274 = flat-sequence {
              tunnel: [w498] -> w493
              tunnel: w493 -> [w500]
              tunnel: [w499] -> w492
              tunnel: w492 -> [w503]
              tunnel: [w502] -> w491
              tunnel: [w501] -> w490
              tunnel: w491 -> [w505]
              tunnel: w490 -> [w504]
              frame #0 {
                n275 = while {
                  stop <- w495 stop-if-true
                  n276 = local read "Z040 RFID"() -> (w497:string)
                  n277 = Wait Until Next ms Multiple(millisecond multiple=u32 50 ("毫秒计时值")) -> ()  [unwired: 1 out]
                  n278 = Not Equal?(x=w497, y="") -> (x != y?=w495:bool)
                }
              }
              frame #1 {
                n279 = local read "Z040 RFID"() -> (w498:string)
                n280 = local write "芯片ID"(w498) -> ()
              }
              frame #2 {
                n281 = call "查询产品ID.vi"("芯片编码"=w500) -> ("产品ID"=w499:string)  [unwired: 8 in, 2 out]
              }
              frame #3 {
                n282 = call "查询上序合格.vi"("产品ID"=w503) -> ("本序已做"=w501:bool, "上序合格"=w502:bool)  [unwired: 8 in, 1 out]
                n283 = local write "产品ID"(w503) -> ()
              }
              frame #4 {
                n284 = local write "上序合格"(w505) -> ()
                n285 = local write "上序完成"(w504) -> ()
              }
              frame #5 {
                n286 = local write "RFID读取完成"(TRUE ("RFID读取完成")) -> ()
                n287 = local write "RFID读取触发"(FALSE ("RFID读取触发")) -> ()
              }
              frame #6 {
                n288 = local write "流水线工步号"(30.0 ("工步号")) -> ()
              }
            }
          }
        }
      }
      frame 600 {
        n289 = flat-sequence {
          tunnel: [w513] -> w509
          tunnel: w509 -> [w524]
          frame #0 {
            n290 = local read "本序合格"() -> (w518:bool)
            n291 = local read "KSJJ"() -> (w517:string)
            n292 = local read "产品ID"() -> (w512:string)
            n293 = local read "员工姓名"() -> (w519:string)
            n294 = Boolean To (0,1)(Boolean=w518) -> (0, 1=w522:i16)
            n295 = Format Date/Time String(time format string (%c)="%Y%m%d%H%M" ("时间格式字符串(%c)")) -> (date/time string=w520:string)  [unwired: 2 in]
            n296 = local read "FGCS"() -> (w515:string)
            n297 = Number To Decimal String(number=w522, width (-)=i16 1 ("宽度(-)")) -> (decimal integer string=w510:string)
            n298 = Build Array(w512, w519, "1" ("元素"), w510, w517, w520, w515, "Q14070-Z040") -> (w513:string[])
          }
          frame #1 {
            n299 = call "数据库更新.vi"("设备号"="04", "数据"=w524) -> ()  [unwired: 13 in, 1 out]
            n300 = Wait (ms)(milliseconds to wait=u32 500 ("等待时间（毫秒）")) -> ()  [unwired: 1 out]
          }
          frame #2 {
            n301 = local write "流水线工步号"(660.0 ("工步号")) -> ()
          }
        }
      }
    }
    n302 = Wait Until Next ms Multiple(millisecond multiple=u32 50 ("毫秒倍数")) -> ()  [unwired: 1 out]
    n303 = local read "停止"() -> (w488:bool)
  }
  n304 = while {
    stop <- w527 stop-if-true
    n305 = stacked-sequence {
      frame #0 {
        n306 = First Call?() -> (First Call?: T/F=w529:bool)
        n307 = case shown="真" w529 {
          frame False {
          }
          frame True {
            n308 = call "员工管理测试程序.vi"() -> ("员工姓名"=w530:string)  [unwired: 11 in]
            n309 = local write "员工姓名"(w530) -> ()
          }
        }
      }
      frame #1 {
        n310 = local read "报警工步号"() -> (w532:dbl)
        n311 = local read "测试 工步号"() -> (w534:dbl)
        n312 = local read "流水线工步号"() -> (w539:dbl)
        n313 = case shown="547" w539 {
          tunnel: [w599 "首先取下装钢球的辅具，准备放钢球" ("工步操作状态") "等待扫描条码" ("工步操作状态") "自动放钢球启动" ("工步操作状态") "判断上序是否合格" ("工步操作状态") "放钢球结束" ("工步操作状态") "补钢球" ("工步操作状态") "上阻挡器放行" ("工步操作状态") "装钢球辅具放回" ("工步操作状态") "取拧紧辅具" ("工步操作状态") "本工位检测" ("工步操作状态") "流水线顶升夹紧" ("工步操作状态") "左标准气缸前进 " ("工步操作状态") "右标准气缸前进" ("工步操作状态") "给出流水线准备好信号" ("工步操作状态") "拧紧辅具放回" ("工步操作状态") "等待测试工位完成信号" ("工步操作状态") "给出本工位完成信号" ("工步操作状态") "右标准气缸回退" ("工步操作状态") "左标准气缸回退" ("工步操作状态") "等待扳手加力" ("工步操作状态") "流水线气缸下降" ("工步操作状态") "流水线顶升气缸下降" ("工步操作状态") "本工位放行" ("工步操作状态") "放行完成" ("工步操作状态") "流水线位动作完成" ("工步操作状态") "上序不合格，则上工位直接放行" ("工步操作状态") "本工位放行" ("工步操作状态") "放行完成" ("工步操作状态") "不合格品，复位解除" ("工步操作状态") "补钢球完成" ("工步操作状态") "循环结束" ("工步操作状态")] -> w538
          frame 0, Default {
            n314 = local read "联线按钮"() -> (w598:bool)
            n315 = case shown="假" w598 {
              tunnel: ["等待工件" ("工步操作状态") "等待扫描条码" ("工步操作状态")] -> w599
              frame False {
              }
              frame True {
              }
            }
          }
          frame 5 {
          }
          frame 10 {
          }
          frame 20 {
          }
          frame 30 {
          }
          frame 40 {
          }
          frame 60 {
          }
          frame 70 {
          }
          frame 80 {
          }
          frame 85 {
          }
          frame 90 {
          }
          frame 95 {
          }
          frame 100 {
          }
          frame 110 {
          }
          frame 120 {
          }
          frame 130 {
          }
          frame 140 {
          }
          frame 520 {
          }
          frame 530 {
          }
          frame 540 {
          }
          frame 545 {
          }
          frame 547 {
          }
          frame 550 {
          }
          frame 560 {
          }
          frame 580 {
          }
          frame 660 {
          }
          frame 700 {
          }
          frame 705 {
          }
          frame 710 {
          }
          frame 800 {
          }
          frame 810 {
          }
          frame 900 {
          }
        }
        "流水线操作状态" <- w538
        n316 = case shown="176" w532 {
          tunnel: ["无报警" ("工步操作状态") "急停按钮被按下" ("工步操作状态") "输入轴电机报警" ("工步操作状态") "旋转电机报警" ("工步操作状态") "放钢球" ("工步操作状态") "放钢球结束" ("工步操作状态") "补钢球" ("工步操作状态") "装钢球气缸下降" ("工步操作状态") "装钢球辅具放回" ("工步操作状态") "取拧紧辅具" ("工步操作状态") "自动拧紧启动" ("工步操作状态") "拧紧气缸下降 " ("工步操作状态") "拧紧机启动" ("工步操作状态") "拧紧气缸退回" ("工步操作状态") "拧紧辅具放回" ("工步操作状态") "测间隙启动" ("工步操作状态") "上测间隙下降" ("工步操作状态") "下测间隙上" ("工步操作状态") "下测间隙回" ("工步操作状态") "判断合格不合格" ("工步操作状态") "上测间隙回" ("工步操作状态") "压铆启动" ("工步操作状态") "增压缸快进" ("工步操作状态") "增压缸增压" ("工步操作状态") "压铆力判断" ("工步操作状态") "增压缸退回" ("工步操作状态") "不合格品，复位解除" ("工步操作状态") "补钢球完成" ("工步操作状态") "循环结束" ("工步操作状态")] -> w531
          frame 0, Default {
          }
          frame 1 {
          }
          frame 2 {
          }
          frame 4 {
          }
          frame 30 {
          }
          frame 40 {
          }
          frame 60 {
          }
          frame 70 {
          }
          frame 80 {
          }
          frame 85 {
          }
          frame 90 {
          }
          frame 100 {
          }
          frame 110 {
          }
          frame 120 {
          }
          frame 130 {
          }
          frame 140 {
          }
          frame 150 {
          }
          frame 160 {
          }
          frame 170 {
          }
          frame 175 {
          }
          frame 176 {
          }
          frame 180 {
          }
          frame 190 {
          }
          frame 200 {
          }
          frame 210 {
          }
          frame 211 {
          }
          frame 800 {
          }
          frame 810 {
          }
          frame 900 {
          }
        }
        "报警信息" <- w531
        n317 = case shown="211" w534 {
          tunnel: ["等待流水线准备好信号" ("工步操作状态") "首先取下装钢球的辅具，准备放钢球" ("工步操作状态") "装钢球气缸顶起" ("工步操作状态") "等待电动缸初始位置完成" ("工步操作状态") "放钢球" ("工步操作状态") "" ("工步操作状态") "" ("工步操作状态") "" ("工步操作状态") "" ("工步操作状态") "" ("工步操作状态") "" ("工步操作状态") "等待输入轴电机初始位置完成 " ("工步操作状态") "" ("工步操作状态") "测试开始" ("工步操作状态") "" ("工步操作状态") "测间隙启动" ("工步操作状态") "测间隙下降" ("工步操作状态") "下测间隙上" ("工步操作状态") "下测间隙回" ("工步操作状态") "判断合格不合格" ("工步操作状态") "上测间隙回" ("工步操作状态") "压铆启动" ("工步操作状态") "增压缸快进" ("工步操作状态") "增压缸增压" ("工步操作状态") "压铆力判断" ("工步操作状态") "增压缸退回" ("工步操作状态") "不合格品，复位解除" ("工步操作状态") "补钢球完成" ("工步操作状态") "循环结束" ("工步操作状态")] -> w533
          frame 0, Default {
          }
          frame 5 {
          }
          frame 10 {
          }
          frame 20 {
          }
          frame 30 {
          }
          frame 40 {
          }
          frame 60 {
          }
          frame 70 {
          }
          frame 80 {
          }
          frame 85 {
          }
          frame 90 {
          }
          frame 100 {
          }
          frame 110 {
          }
          frame 120 {
          }
          frame 130 {
          }
          frame 140 {
          }
          frame 150 {
          }
          frame 160 {
          }
          frame 170 {
          }
          frame 175 {
          }
          frame 176 {
          }
          frame 180 {
          }
          frame 190 {
          }
          frame 200 {
          }
          frame 210 {
          }
          frame 211 {
          }
          frame 800 {
          }
          frame 810 {
          }
          frame 990 {
          }
        }
        "测试操作状态" <- w533
        n318 = local read "输入轴AxisHandle OUT"() -> (w535:u32)
        n319 = call <userlib>:"Acm_AxDiGetBit.vi"("DiChannel"=u16 3, "AxisHandle"=w535) -> ("ReturnValue"=→"ReturnValue 3":u32)  [unwired: 2 in, 3 out]
      }
      frame #2 {
        n320 = local read "力矩（nm)"() -> (w638:dbl)
        n321 = local read "电机下降"() -> (w640:bool)
        n322 = local read "电机上升"() -> (w639:bool)
        n323 = Absolute Value(x=w638) -> (abs(x)=w637:dbl)
        n324 = Not(x=w639) -> (.not. x?=w635:bool)
        n325 = Less?(x=w637, y=20.0) -> (x < y?=w634:bool)
        n326 = Compound Arithmetic op=AND(w640, w635, w634) -> (w633:bool)
        n327 = case shown="真" w633 {
          frame False {
          }
          frame True {
            n328 = flat-sequence {
              tunnel: [w647] -> w642
              tunnel: w642 -> [w650]
              tunnel: [w650] -> w641
              tunnel: w641 -> [w651]
              tunnel: [w651] -> w643
              tunnel: w643 -> [w663]
              frame #0 {
                n329 = local read "输入轴AxisHandle OUT"() -> (w645:u32)
                n330 = call "PCI1220U使能.vi"("使能"=TRUE, "AxisHandle IN"=w645) -> ()  [unwired: 9 in, 1 out]
              }
              frame #1 {
                n331 = local write "进给速度"(5.0 ("进给速度")) -> ()
              }
              frame #2 {
                n332 = local read "输入轴AxisHandle OUT"() -> (w649:u32)
                n333 = call "PCI1220U运行.vi"("方向"=u16 0, "AxisHandle IN"=w649) -> ("AxisHandle OUT"=w647:u32)  [unwired: 9 in]
              }
              frame #3 {
              }
              frame #4 {
                n334 = while {
                  stop <- w655 stop-if-true
                  n335 = local read "力矩（nm)"() -> (w658:dbl)
                  n336 = local read "急停按钮"() -> (w654:bool)
                  n337 = local read "复位按钮"() -> (w652:bool)
                  n338 = local read "电机下降"() -> (w662:bool)
                  n339 = Absolute Value(x=w658) -> (abs(x)=w659:dbl)
                  n340 = Greater Or Equal?(x=w659, y=20.0) -> (x >= y?=w656:bool)
                  n341 = Not(x=w654) -> (.not. x?=w653:bool)
                  n342 = Not(x=w662) -> (.not. x?=w657:bool)
                  n343 = Wait Until Next ms Multiple(millisecond multiple=u32 50 ("毫秒倍数")) -> ()  [unwired: 1 out]
                  n344 = Compound Arithmetic op=OR(w657, w656, w653, w652) -> (w655:bool)
                }
              }
              frame #5 {
                n345 = call "PCI1220U停止.vi"("AxisHandle IN"=w663) -> ()  [unwired: 9 in, 2 out]
              }
            }
          }
        }
      }
      frame #3 {
        n346 = local read "力矩（nm)"() -> (w671:dbl)
        n347 = local read "电机上升"() -> (w665:bool)
        n348 = local read "电机下降"() -> (w664:bool)
        n349 = Absolute Value(x=w671) -> (abs(x)=w670:dbl)
        n350 = Not(x=w664) -> (.not. x?=w668:bool)
        n351 = Less?(x=w670, y=20.0) -> (x < y?=w667:bool)
        n352 = Compound Arithmetic op=AND(w665, w668, w667) -> (w666:bool)
        n353 = case shown="真" w666 {
          frame False {
          }
          frame True {
            n354 = flat-sequence {
              tunnel: [w678] -> w674
              tunnel: w674 -> [w681]
              tunnel: [w681] -> w673
              tunnel: w673 -> [w682]
              tunnel: [w682] -> w672
              tunnel: w672 -> [w695]
              frame #0 {
                n355 = local read "输入轴AxisHandle OUT"() -> (w676:u32)
                n356 = call "PCI1220U使能.vi"("使能"=TRUE, "AxisHandle IN"=w676) -> ()  [unwired: 9 in, 1 out]
              }
              frame #1 {
                n357 = local write "进给速度"(5.0 ("进给速度")) -> ()
              }
              frame #2 {
                n358 = local read "输入轴AxisHandle OUT"() -> (w680:u32)
                n359 = call "PCI1220U运行.vi"("方向"=u16 1, "AxisHandle IN"=w680) -> ("AxisHandle OUT"=w678:u32)  [unwired: 9 in]
              }
              frame #3 {
              }
              frame #4 {
                n360 = while {
                  stop <- w691 stop-if-true
                  n361 = local read "力矩（nm)"() -> (w687:dbl)
                  n362 = local read "电机上升"() -> (w690:bool)
                  n363 = local read "急停按钮"() -> (w685:bool)
                  n364 = local read "复位按钮"() -> (w683:bool)
                  n365 = Absolute Value(x=w687) -> (abs(x)=w688:dbl)
                  n366 = Not(x=w690) -> (.not. x?=w692:bool)
                  n367 = Greater Or Equal?(x=w688, y=20.0) -> (x >= y?=w686:bool)
                  n368 = Not(x=w685) -> (.not. x?=w684:bool)
                  n369 = Wait Until Next ms Multiple(millisecond multiple=u32 50 ("毫秒倍数")) -> ()  [unwired: 1 out]
                  n370 = Compound Arithmetic op=OR(w692, w686, w684, w683) -> (w691:bool)
                }
              }
              frame #5 {
                n371 = call "PCI1220U停止.vi"("AxisHandle IN"=w695) -> ()  [unwired: 9 in, 2 out]
                n372 = Wait (ms)(milliseconds to wait=u32 100 ("毫秒计时值")) -> ()  [unwired: 1 out]
              }
            }
          }
        }
      }
      frame #4 {
        n373 = local read "右旋"() -> (w696:bool)
        n374 = local read "力矩（nm)"() -> (w703:dbl)
        n375 = local read "左旋"() -> (w697:bool)
        n376 = Absolute Value(x=w703) -> (abs(x)=w702:dbl)
        n377 = Not(x=w696) -> (.not. x?=w700:bool)
        n378 = Less?(x=w702, y=20.0) -> (x < y?=w699:bool)
        n379 = Compound Arithmetic op=AND(w697, w700, w699) -> (w698:bool)
        n380 = case shown="真" w698 {
          frame False {
          }
          frame True {
            n381 = flat-sequence {
              tunnel: [w709] -> w704
              tunnel: [w711] -> w705
              tunnel: w704 -> [w711]
              tunnel: [w714] -> w708
              tunnel: w705 -> [w713]
              tunnel: w708 -> [w716]
              tunnel: [w716] -> w707
              tunnel: w707 -> [w717]
              tunnel: [w717] -> w706
              tunnel: w706 -> [w730]
              frame #0 {
                n382 = local read "旋转轴AxisHandle OUT"() -> (w709:u32)
                n383 = call "PCI1220U使能.vi"("使能"=TRUE, "AxisHandle IN"=w709) -> ()  [unwired: 9 in, 1 out]
              }
              frame #1 {
                n384 = local write "旋转速度"(10.0 ("进给速度")) -> ()
              }
              frame #2 {
                n385 = call "PCI1220U运行.vi"("方向"=u16 0, "AxisHandle IN"=w713) -> ("AxisHandle OUT"=w714:u32)  [unwired: 9 in]
              }
              frame #3 {
              }
              frame #4 {
                n386 = while {
                  stop <- w726 stop-if-true
                  n387 = local read "力矩（nm)"() -> (w723:dbl)
                  n388 = local read "急停按钮"() -> (w721:bool)
                  n389 = local read "左旋"() -> (w718:bool)
                  n390 = local read "复位按钮"() -> (w719:bool)
                  n391 = Absolute Value(x=w723) -> (abs(x)=w724:dbl)
                  n392 = Not(x=w718) -> (.not. x?=w727:bool)
                  n393 = Greater Or Equal?(x=w724, y=20.0) -> (x >= y?=w722:bool)
                  n394 = Not(x=w721) -> (.not. x?=w720:bool)
                  n395 = Wait Until Next ms Multiple(millisecond multiple=u32 50 ("毫秒倍数")) -> ()  [unwired: 1 out]
                  n396 = Compound Arithmetic op=OR(w727, w722, w720, w719) -> (w726:bool)
                }
              }
              frame #5 {
                n397 = call "PCI1220U停止.vi"("AxisHandle IN"=w730) -> ()  [unwired: 9 in, 2 out]
                n398 = Wait (ms)(milliseconds to wait=u32 100 ("毫秒计时值")) -> ()  [unwired: 1 out]
              }
            }
          }
        }
      }
      frame #5 {
        n399 = local read "力矩（nm)"() -> (w738:dbl)
        n400 = local read "右旋"() -> (w732:bool)
        n401 = local read "左旋"() -> (w731:bool)
        n402 = Absolute Value(x=w738) -> (abs(x)=w737:dbl)
        n403 = Not(x=w731) -> (.not. x?=w735:bool)
        n404 = Less?(x=w737, y=20.0) -> (x < y?=w734:bool)
        n405 = Compound Arithmetic op=AND(w732, w735, w734) -> (w733:bool)
        n406 = case shown="真" w733 {
          frame False {
          }
          frame True {
            n407 = flat-sequence {
              tunnel: [w744] -> w739
              tunnel: [w747] -> w740
              tunnel: w739 -> [w747]
              tunnel: [w749] -> w743
              tunnel: w740 -> [w748]
              tunnel: w743 -> [w751]
              tunnel: [w751] -> w742
              tunnel: w742 -> [w752]
              tunnel: [w752] -> w741
              tunnel: w741 -> [w765]
              frame #0 {
                n408 = local read "旋转轴AxisHandle OUT"() -> (w744:u32)
                n409 = call "PCI1220U使能.vi"("使能"=TRUE, "AxisHandle IN"=w744) -> ()  [unwired: 9 in, 1 out]
              }
              frame #1 {
                n410 = local write "旋转速度"(10.0 ("进给速度")) -> ()
              }
              frame #2 {
                n411 = call "PCI1220U运行.vi"("方向"=u16 1, "AxisHandle IN"=w748) -> ("AxisHandle OUT"=w749:u32)  [unwired: 9 in]
              }
              frame #3 {
              }
              frame #4 {
                n412 = while {
                  stop <- w761 stop-if-true
                  n413 = local read "力矩（nm)"() -> (w758:dbl)
                  n414 = local read "右旋"() -> (w753:bool)
                  n415 = local read "急停按钮"() -> (w756:bool)
                  n416 = local read "复位按钮"() -> (w754:bool)
                  n417 = Absolute Value(x=w758) -> (abs(x)=w759:dbl)
                  n418 = Not(x=w753) -> (.not. x?=w762:bool)
                  n419 = Greater Or Equal?(x=w759, y=20.0) -> (x >= y?=w757:bool)
                  n420 = Not(x=w756) -> (.not. x?=w755:bool)
                  n421 = Wait Until Next ms Multiple(millisecond multiple=u32 50 ("毫秒倍数")) -> ()  [unwired: 1 out]
                  n422 = Compound Arithmetic op=OR(w762, w757, w755, w754) -> (w761:bool)
                }
              }
              frame #5 {
                n423 = call "PCI1220U停止.vi"("AxisHandle IN"=w765) -> ()  [unwired: 9 in, 2 out]
                n424 = Wait (ms)(milliseconds to wait=u32 100 ("毫秒计时值")) -> ()  [unwired: 1 out]
              }
            }
          }
        }
      }
    }
    n425 = Wait Until Next ms Multiple(millisecond multiple=u32 50 ("毫秒倍数")) -> ()  [unwired: 1 out]
    n426 = local read "停止"() -> (w527:bool)
  }
  n427 = flat-sequence {
    tunnel: [w767] -> w6
    tunnel: [w766] -> w5
    tunnel: w6 -> [w774]
    tunnel: w5 -> [w773]
    tunnel: [w772] -> w4
    tunnel: [w771] -> w3
    tunnel: w4 -> [w873]
    tunnel: w3 -> [w872]
    frame #0 {
      n428 = call "ADO Connection Create.vi"() -> ("error out"=w769:errorcluster, "ADODB._Connection Out"=w770:refnum<k7>)  [unwired: 10 in]
      n429 = call "ADO Connection Open.vi"("error in (no error)"=w769, "ConnectionString"="DSN=参数Z040;", "ADODB._Connection In"=w770) -> ("error out"=w766:errorcluster, "ADODB._Connection Out"=w767:refnum<k7>)  [unwired: 7 in]
      "ADODB._Connection Out" <- w767
    }
    frame #1 {
      n430 = while {
        tunnel: w774 -> [w779]
        tunnel: w773 -> [w778]
        tunnel: [w777] -> w772
        tunnel: [w776] -> w771
        stop <- w782 stop-if-true
        n431 = local read "参数加载"() -> (w775:bool)
        n432 = Wait (ms)(milliseconds to wait=u32 200 ("等待时间（毫秒）")) -> ()  [unwired: 1 out]
        n433 = First Call?() -> (First Call?: T/F=w781:bool)
        n434 = Or(x=w781, y=w775) -> (x .or. y?=w780:bool)
        n435 = case shown="真" w780 {
          tunnel: w779 -> [w785 w789]
          tunnel: w778 -> [w784 w788]
          tunnel: [w785 w787] -> w777
          tunnel: [w784 w786] -> w776
          frame False {
          }
          frame True {
            n436 = stacked-sequence {
              seq-local: [w793 _ _] -> [_ w856 _]
              tunnel: w789 -> [w794 w853 _]
              tunnel: w788 -> [w795 _ _]
              tunnel: [w794 _ _] -> w787
              tunnel: [_ w855 _] -> w786
              frame #0 {
                n437 = First Call?() -> (First Call?: T/F=w792:bool)
                n438 = local read "参数加载"() -> (w791:bool)
                n439 = Or(x=w792, y=w791) -> (x .or. y?=w790:bool)
                n440 = case shown="真" w790 {
                  tunnel: w795 -> [w796 w801]
                  tunnel: w794 -> [_ w799]
                  tunnel: [w796 w798] -> w793
                  frame False {
                  }
                  frame True {
                    n441 = call "SQL Execute.vi"("error in (no error)"=w801, "Command Text"="SELECT * FROM 测试参数表 ;", "ADODB._Connection In"=w799) -> ("error out"=w798:errorcluster, "Data"=w802:string[][])  [unwired: 5 in, 2 out]
                    n442 = Index Array "索引数组"(array=w802, index (col)=0 ("禁用的索引 (列)")) -> (element=w805:string[])  [unwired: 1 in]
                    n443 = Array Size "数组大小"(array=w805) -> (size(s)=w804:i32)
                    n444 = while {
                      shift-right: [w810] -> w803
                      shift-left: i32[] [] -> [w811]
                      tunnel: w804 -> [w808]
                      i -> [w809]
                      stop <- w812 stop-if-true
                      n445 = Greater Or Equal?(x=w809, y=w808) -> (x >= y?=w812:bool)
                      n446 = Build Array (concatenate) "创建数组"(w811, w809) -> (w810:i32[])
                    }
                    n447 = Build Cluster Array "索引与捆绑簇数组"(w805, w803) -> (w797:cluster{"String":string, i32}[])
                    n448 = property on="型号选择" class="Ring (严格)"("StringsAndValues[]"=w797) -> ()  [unwired: 2 in, 2 out]
                  }
                }
              }
              frame #1 {
                (unwired) ",产品型号,输入轴电机快进位置,输入轴电机快进速度,输入轴电机慢进位置,输入轴电机慢进速度,旋转电机位置1,旋转电机位置2,旋转电机速度,换向扭矩,间隙判定值" ("查询内容")
                n449 = property on="型号选择" class="Ring (严格)"() -> ("RingText.Text"=w852:string)  [unwired: 2 in, 2 out]
                n450 = call "创建文本3"("产品型号"=w852) -> ("Result"=w854:string)  [unwired: 13 in, 1 out]
                n451 = call "SQL Execute.vi"("error in (no error)"=w856, "Command Text"=w854, "ADODB._Connection In"=w853) -> ("error out"=w855:errorcluster, "Data"=w858:string[][])  [unwired: 5 in, 2 out]
                n452 = Index Array "索引数组"(array=w858, index (row)=0 ("索引 (行)")) -> (element=w851:string[])  [unwired: 1 in]
                n453 = Fract/Exp String To Number "分数/指数字符串至数值转换"(string=w851) -> (number=w825:dbl[])  [unwired: 3 in, 1 out]
                n454 = Index Array(array=w825, index #1=1 ("索引"), index #2=2 ("索引"), index #3=3 ("索引"), index #4=4 ("索引"), index #5=5 ("索引"), index #6=6 ("索引"), index #7=7 ("索引"), index #8=8 ("索引"), index #9=9 ("索引"), index #10=10 ("索引"), index #11=11 ("索引"), index #12=12 ("索引"), index #13=13 ("索引"), index #14=14 ("索引"), index #15=15 ("索引"), index #16=16 ("索引"), index #17=17 ("索引"), index #18=18 ("索引"), index #19=19 ("索引"), index #20=20 ("索引"), index #21=21 ("索引"), index #22=22 ("索引"), index #23=23 ("索引"), index #24=24 ("索引")) -> (element #1=w824:dbl, element #2=→"输入轴电机快进速度":dbl, element #3=w823:dbl, element #4=→"输入轴电机慢进位置2":dbl, element #5=→"输入轴电机慢进位置3":dbl, element #6=→"输入轴电机慢进速度":dbl, element #7=→"输入轴最终位置（mm)":dbl, element #8=w818:dbl, element #9=w817:dbl, element #10=→"旋转电机速度":dbl, element #11=w815:dbl, element #12=w814:dbl, element #13=w813:dbl)  [unwired: 11 out]
                n455 = local write "间隙合格标准值(mm)"(w813) -> ()
                n456 = local write "输入轴快进位置(mm)"(w824) -> ()
                n457 = local write "旋转左极限位(mm)"(w818) -> ()
                n458 = local write "旋转右极限位(mm)"(w817) -> ()
                n459 = local write "换向扭矩(NM)"(w815) -> ()
                n460 = local write "检测扭矩(NM)"(w814) -> ()
                n461 = local write "输入轴初始位置(mm)"(w823) -> ()
              }
              frame #2 {
                n462 = local read "ADODB._Connection Out"() -> (w866:refnum<k7>)
                n463 = call "SQL Execute.vi"("Command Text"="SELECT * FROM 传感器校验表 where ID='2'", "ADODB._Connection In"=w866) -> ("Data"=w871:string[][])  [unwired: 6 in, 3 out]
                n464 = Index Array "索引数组"(array=w871) -> (element=w870:string[])  [unwired: 2 in]
                n465 = Fract/Exp String To Number "分数/指数字符串至数值转换"(string=w870) -> (number=w869:dbl[])  [unwired: 3 in, 1 out]
                n466 = Index Array "索引数组"(array=w869, index #1=1 ("索引"), index #2=2 ("索引"), index #3=3 ("索引"), index #4=4 ("索引")) -> (element #1=w862:dbl, element #2=w861:dbl, element #3=w860:dbl, element #4=w859:dbl)
                n467 = local write "扭矩传感器零点偏移"(w862) -> ()
                n468 = local write "扭矩传感器比例偏移"(w861) -> ()
                n469 = local write "位移传感器零点偏移"(w860) -> ()
                n470 = local write "位移传感器比例偏移"(w859) -> ()
              }
            }
          }
        }
        n471 = local read "停止"() -> (w782:bool)
      }
    }
    frame #2 {
      n472 = call "ADO Connection Close.vi"("error in (no error)"=w872, "ADODB._Connection In"=w873) -> ("error out"=→"error out 2":errorcluster)  [unwired: 8 in, 1 out]
    }
  }
  n473 = flat-sequence {
    tunnel: [w878] -> w9
    tunnel: [w876] -> w2
    tunnel: [w875] -> w1
    tunnel: w9 -> [w882]
    tunnel: [w881] -> w8
    tunnel: w2 -> [w880]
    tunnel: w1 -> [w879]
    tunnel: w8 -> [w936]
    tunnel: [w936] -> w7
    tunnel: w7 -> [w938]
    frame #0 {
      n474 = call "PCI1240U初始化.vi"() -> ("2电机"=w875:u32, "1电机"=w876:u32, "DeviceHandle"=→"DeviceHandle":u32)  [unwired: 6 in, 3 out]
      "输入轴AxisHandle OUT" <- w875
      "旋转轴AxisHandle OUT" <- w876
      n475 = call "PCI8622配置.vi"() -> ("DeviceID"=w878:i32)  [unwired: 11 in]
    }
    frame #1 {
      n476 = while {
        tunnel: w882 -> [w922]
        tunnel: [w922] -> w881
        tunnel: w880 -> [w884]
        tunnel: w879 -> [w883]
        stop <- "停止" stop-if-true
        w932 = 0  # nRetSizeWords
        w933 = 2048  # nReadSizeWords
        # "hDevice"
        n477 = Wait Until Next ms Multiple(millisecond multiple=u32 50 ("毫秒倍数")) -> ()  [unwired: 1 out]
        n478 = Initialize Array(u16 0, 2048 ("dimension size")) -> (w923:u16[])
        n479 = dll-call lib="PCI8622_32.dll" fn="PCI8622_ReadDeviceProAD_Npt" label="ReadDeviceProAD_Npt"("hDevice"=w922, "ADBuffer[]"=w923, "nReadSizeWords"=w933, "nRetSizeWords"=w932) -> ("ADBuffer[]"=w926:u16[])  [unwired: 7 in, 2 out]
        n480 = Divide(x=w926, y=65536.01) -> (x/y=w927:dbl[])
        n481 = Multiply(x=w927, y=20) -> (x*y=w930:dbl[])
        n482 = call "PCI1220U速度设置.vi"("Change Velocity"="旋转速度", "AxisHandle IN"=w884) -> ("AxisHandle OUT"=w888:u32)  [unwired: 9 in]
        n483 = call "PCI1220电动缸速度设置.vi"("Change Velocity"="进给速度", "AxisHandle IN"=w883) -> ("AxisHandle OUT"=w887:u32)  [unwired: 8 in]
        n484 = Subtract(x=w930, y=10) -> (x-y=w918:dbl[])
        n485 = Decimate 1D Array "抽取一维数组"(w918) -> (w895:dbl[], w894:dbl[])  [unwired: 6 out]
        n486 = call "PCI1220电动缸读取位置.vi"("AxisHandle IN"=w887) -> ("位置"=→"输入轴伺服位置":dbl)  [unwired: 9 in, 1 out]
        n487 = Add Array Elements(numeric array=w894) -> (sum=w907:dbl)
        n488 = Add Array Elements(numeric array=w895) -> (sum=w920:dbl)
        n489 = Array Size(array=w894) -> (size(s)=w906:i32)
        n490 = Array Size(array=w895) -> (size(s)=w919:i32)
        n491 = Divide(x=w907, y=w906) -> (x/y=w905:dbl)
        n492 = Divide(x=w920, y=w919) -> (x/y=w916:dbl)
        n493 = call "PCI1220U读取位置.vi"("AxisHandle IN"=w888) -> ("位置"=→"旋转轴伺服位置":dbl)  [unwired: 9 in, 1 out]
        n494 = local read "位移传感器零点偏移"() -> (w898:dbl)
        n495 = local read "扭矩传感器零点偏移"() -> (w909:dbl)
        n496 = local read "位移传感器比例偏移"() -> (w896:dbl)
        n497 = Subtract(x=w905, y=3.7) -> (x-y=w903:dbl)
        n498 = Subtract(x=w916, y=-0.0) -> (x-y=w915:dbl)
        n499 = Multiply(x=w903, y=1.0) -> (x*y=w901:dbl)
        n500 = Multiply(x=w915, y=5.0) -> (x*y=w913:dbl)
        n501 = local read "扭矩传感器比例偏移"() -> (w908:dbl)
        n502 = Subtract(x=w901, y=0.0) -> (x-y=w899:dbl)
        n503 = Subtract(x=w913, y=0.0) -> (x-y=w912:dbl)
        n504 = Subtract(x=w899, y=w898) -> (x-y=w897:dbl)
        n505 = Subtract(x=w912, y=w909) -> (x-y=w911:dbl)
        n506 = Multiply(x=w897, y=w896) -> (x*y=w893:dbl)
        n507 = Multiply(x=w911, y=w908) -> (x*y=→"力矩（nm)":dbl)
        n508 = call "滤波器"("Signal"=w893) -> ("Filtered Signal"=→"位移(mm)":dynamicdata)  [unwired: 9 in, 1 out]
      }
    }
    frame #2 {
      n509 = dll-call lib="PCI8622_32.dll" fn="PCI8622_StopDeviceProAD" label="StopDeviceProAD"("hDevice"=w936) -> ("hDevice"=w937:i32)  [unwired: 4 in, 2 out]
      n510 = local read "DeviceHandle"() -> (w935:u32)
      n511 = dll-call lib="PCI8622_32.dll" fn="PCI8622_ReleaseDeviceProAD" label="ReleaseDeviceProAD"("hDevice"=w937) -> ()  [unwired: 5 in, 2 out]
      n512 = call <userlib>:"Acm_DevClose.vi"("DeviceHandle"=w935) -> ()  [unwired: 1 in, 2 out]
    }
    frame #3 {
      n513 = dll-call lib="PCI8622_32.dll" fn="PCI8622_ReleaseDevice" label="ReleaseDevice"("hDevice"=w938) -> ()  [unwired: 5 in, 2 out]
    }
  }
